vi "MainN.vi"() -> ()   [LabVIEW 2013]
uses:
  ReceiveStrDismantle/MMI_BCM_2A1.ctl
  ReceiveStrDismantle/MMI_AC_2.ctl
  ReceiveStrDismantle/MMI_PEPS_2A7.ctl
  Log.ctl
  SendCmdStr/Input1.ctl
  SendCmdStr/Input2.ctl
  SendCmdStr/HVSM.ctl
  SendCmdStr/TCM.ctl
  SendCmdStr/AC_2F1.ctl
  SendCmdStr/AC_2F2.ctl
  SendCmdStr/BCM_284.ctl
  SendCmdStr/BCM_LDoor_285.ctl
  SendCmdStr/BCM_287.ctl
  SendCmdStr/GW_PEPS_2FC.ctl
  SendCmdStr/TCU_113.ctl
  SendCmdStr/ESC_125.ctl
  SendCmdStr/SAS_0E0.ctl
  SendCmdStr/BCM_Ligh_1F0.ctl
  SendCmdStr/IPK_3F0.ctl
  GlobalVariable.vi
  CAN/ControlCAN.dll
panel:
  in  "刷新":bool
  in  "周期":u32=100
  out "LogEvent":refnum<user-event>
  in  "Input2":T1
  in  "Input1":T2
  in  "Log":T3
  out "消息":string
  in  "接收":bool
  in  "arraylen":u32
  in  "TREvent":T4={"Tx_Or_Rx"=FALSE, "VCI_CAN_OBJ"={"ID"=0, "TimeStamp"=0, "TimeFlag"=0, "SendType"=1, "RemoteFlag"=0, "ExternFlag"=0, "DataLen"=8, 0, 0, 0, 0, 0, 0, 0, 0, 0, 0, 0}, "VCI_CAN_OBJ_N"=[], "Num"=0}
  out "VCI_CAN_STATUS":T5
  in  "界面标识":string="显示界面"
  in  "滤波ID":u32 format="0x%08x"
  in  "滤波":bool
  in  "发送 ID":u32 format="0x%08x"
  in  "一次发送帧数":u32=1
  out "接收缓冲区":u32
  in  "GetStatus":bool
  in  "GetErrorInfo":bool
  in  "Clear Buffer":bool
  in  "Transmit":bool
  in  "数据输入":string
  in  "帧格式":u8(ring) items=["数据帧", "远程帧"]
  in  "帧类型":u8(ring) items=["标准帧", "扩展帧"]
  in  "发送类型":u8(ring) items=["正常发送", "单次发送", "自发自收", "单次自发自收"]
  in  "索引":u32(ring) items=["0", "1", "2", "3", "4", "5", "6", "7", "8"]
  out "CANStartup":bool
  in  "DevOpen":bool
  in  "OpenDevice":bool
  in  "设备类型":u32(ring)=3 items=["PCI5121"=1, "PCI9810"=2, "USBCAN1"=3, "USBCAN2"=4, "PCI9820"=5, "PCI5110"=7, "PC104CAN"=11, "CANETUDP"=12, "PCI9840B"=14, "PC104C2"=15, "PCI9820I"=16, "CANETTCP"=17, "PCIE9221"=24]
  in  "ResetCAN":bool
  in  "StartCAN":bool
  in  "CAN 通道":u32(ring) items=["0", "1"]
  in  "Baud":u32(ring)=11 caption="波特率" items=["5Kbps", "10Kbps", "20Kbps", "40Kbps", "50Kbps", "80Kbps", "100Kbps", "125Kbps", "200Kbps", "250Kbps", "400Kbps", "500Kbps", "666Kbps", "800Kbps", "1000Kbps"]
  in  "模式":u8(ring) items=["正常", "只听"]
  in  "滤波方式":u8(ring)=1 items=["双滤波", "单滤波"]
  in  "BTR1":u8=20 format="0x%02x"
  in  "BTR0":u8 format="0x%02x"
  in  "屏蔽码":u32=4294967295 format="0x%08x"
  in  "验收码":u32 format="0x%08x"
  out "VCI_ERR_INFO":T6 {"ArLost_ErrData" format="%.0x"; "Passive_ErrData2" format="%.0x"; "Passive_ErrData1" format="%.0x"; "Passive_ErrData0" format="%.0x"; "ErrCode" format="%.0x"}
  out "VCI_CAN_OBJ_TN":T7(array[cluster])
  out "VCI_CAN_OBJ_RN":T7(array[cluster])
  out "VCI_INIT_CONFIG":T8={"AccCode"=0, "AccMask"=4294967295, "Reserved"=0, "Filter"=1, "Timing0"=0, "Timing1"=20, "Mode"=0}
  out "VCI_CAN_OBJ_T":T9={"ID"=0, "TimeStamp"=0, "TimeFlag"=0, "SendType"=1, "RemoteFlag"=0, "ExternFlag"=0, "DataLen"=8, 0, 0, 0, 0, 0, 0, 0, 0, 0, 0, 0}
  out "VCI_CAN_OBJ_R":T9={"ID"=0, "TimeStamp"=0, "TimeFlag"=0, "SendType"=1, "RemoteFlag"=0, "ExternFlag"=0, "DataLen"=8, 0, 0, 0, 0, 0, 0, 0, 0, 0, 0, 0}
  in  "多列列表框":i32(listbox)
  in  "退出":bool
  in  "前面板显示":enum32{"接收", "发送", "帮助"}(tab)
  in  "显示信息":T10(tab)
  out "GPS位置信息2":T11
  out "时间显示":string="时间显示"
  out "日":dbl
  out "月":dbl
  out "年":dbl
  out "秒":dbl
  out "分":dbl
  out "时":dbl
  out "GPS位置信息1":T11
  out "BCM":T12 {"语音命令天窗开关" items=["默认", "停止"]; "天窗开度" scale=0.0..100.0; "右后侧车窗开度" scale=0.0..100.0; "左后侧车窗开度" scale=0.0..100.0; "副驾驶侧车窗开度" scale=0.0..100.0; "伴我回家时间" items=["无", "30s", "60s", "90s"]; "门解锁设置应答" items=["无应答", "应答驾驶门解锁", "应答所有门解锁"]; "天窗翘起控制" items=["无", "倾斜翘起", "倾斜关闭"]; "车窗防夹报警" items=["无", "禁止", "启用"]; "日间行车灯" items=["无", "禁止", "启用"]; "智能弯道灯" items=["无", "禁止", "启用"]; "后视镜自动折叠" items=["无", "禁止", "启用"]; "下雨关窗模式" items=["无", "关", "开"]; "设防提示类型" items=["无", "亮灯并鸣笛", "亮灯", "鸣笛"]; "驾驶侧车窗开度" scale=0.0..100.0}
  out "AC空调":T13 {"空气质量弹窗提醒" items=["未按下", "取消提醒"]; "吹风模式请求" items=["Face", "Bilevel", "Foot", "Foot Screen", "Screen", "未设置"]; "鼓风机风速档位" items=["关闭", "风速1", "风速2", "风速3", "风速4", "风速5", "风速6", "风速7", "风速8", "未设置"]; "左侧设定温度显示" scale=17.5..31.5; "驻车空调设置" items=["无", "关闭", "开启"]}
  out "Skin":T14 {"SVA声音报警设置" items=["无请求", "禁止", "启用"]; "IPK-HUD-MMI皮肤联动" items=["联动", "未联动"]; "总里程清零命令" items=["无命令", "清零"]; "指示目的地距离单位" items=["无显示", "Meter", "KiloMeter"]; "MMI激活HUD" items=["无", "未激活", "已激活"]; "皮肤模式" items=["皮肤1", "皮肤2", "皮肤3"]; "方向盘多功能开关模式" items=["MMImode", "IPKmode", "HUDmode"]; "方向盘返回键动作" items=["未按下", "短按", "长按", "长按不松手"]; "方向盘确认键动作" items=["未按下", "短按", "长按", "长按不松手"]; "方向盘下指示键动作" items=["未按下", "短按", "长按", "长按不松手"]; "方向盘上指示键动作" items=["未按下", "短按", "长按", "长按不松手"]; "方向盘左指示键动作" items=["未按下", "短按", "长按", "长按不松手"]; "方向盘右指示键动作" items=["未按下", "短按", "长按", "长按不松手"]}
  out "PEPS":T15 {"任意门开启锁车报警" items=["无请求", "禁止", "启用", "预留"]; "天窗/遮阳帘关闭设置" items=["无请求", "天窗关闭", "遮阳帘关闭", "预留"]; "车窗透气开启设置" items=["无请求", "禁止", "启用", "预留"]; "前雨刮激活后雨刮" items=["无请求", "不激活", "激活", "预留"]; "AVM道路中标定请求" items=["无请求", "开始标定", "预留"]; "自动开关窗设置显示" items=["无请求", "RKE长按控制", "车钥匙控制", "预留"]; "迎宾灯功能开关" items=["无请求", "禁止", "启用", "预留"]; "钥匙忘车内锁车报警" items=["无请求", "禁止", "启用", "预留"]; "AVAS禁用设置" items=["无请求", "禁止", "启用", "预留"]; "电源非OFF锁车报警" items=["无请求", "禁止", "启用", "预留"]; "外后视镜倒车倾斜" items=["无请求", "禁止所有倾斜", "启用驾驶侧", "启用乘客侧", "启用所有侧"]}
  out "智能信号管理":T16 {"下一拥堵路段的长度" scale=0.0..100.0; "距离下一拥堵路段距离" scale=0.0..100.0; "下一路段拥堵等级" items=["正常", "等级1", "等级2", "等级3"]; "当前路段拥堵等级" items=["正常", "等级1", "等级2", "等级3"]; "当前行驶路况" items=["普通路况", "高速路况", "其它"]; "当前拥堵路段剩余长度" scale=0.0..100.0}
  out "PAS_FCS":T17 {"EVA与驾驶模式联动" items=["无联动", "联动", "预留"]; "EVA排气声浪开关" items=["无响应", "开", "关", "预留"]; "iBooster制动模式" items=["NoRequest", "ComfortMode", "SportMode ", "预留"]; "SUM与驾驶模式联动选择" items=["无联动", "联动", "预留"]; "SUM模式选择" items=["No Action", "Confort", "Sport", "预留"]; "泊入功能选择" items=["无按键按下", "水平按下", "垂直按下", "预留"]; "PAS-APA功能确认或关闭" items=["无按键按下", "确认键按下", "终止键按下", "预留"]; "泊入泊出功能选择" items=["未按下", "PSC按下", "POC按下", "预留"]; "环视摄像头功能状态" items=["未激活", "激活", "保持", "失败"]; "导航状态" items=["正常", "失败", "预留"]; "当前所处道路类型" items=["未知", "高速路", "乡道", "国道", "省道", "主干道", "分叉路", "其它"]; "来自地图数据库的限速" scale=0.0..255.0; "前方匝道距离" items=["无匝道", "1000m", "500m", "200m", "预留"]}
  in  "动作输出":T18(tab)
  in  "日":u8
  in  "月":u8
  in  "年":u32
  in  "秒":u8
  in  "分":u8
  in  "时":u8
  in  "时间显示制":u16(ring) items=["24h", "12h"]
  out "时间设置":string="时间设置"
  in  "设置时间":bool
  in  "HVSM远程控制模式与否":bool
  in  "副驾座椅加热状态":u8(ring) items=["关闭", "Level1", "Level2", "Level3", "预留", "错误"]
  in  "司机座椅加热状态":u8(ring) items=["关闭", "Level1", "Level2", "Level3", "预留", "错误"]
  in  "仪表显示档位状态":u16(ring) items=["无显示", "显示P", "显示R", "显示N", "显示D", "显示M1", "显示M2", "显示M3", "显示M4", "显示M5", "显示M6", "显示M7", "显示M1+", "显示M2+", "显示M3+", "显示M4+", "显示M5+", "显示M6+", "显示M2-", "显示M3-", "显示M4-", "显示M5-", "显示M6-", "显示M7-", "无效", "预留"]
  in  "TCU档位模式":u16(ring) items=["未定义", "P", "R", "N", "D", "M", "预留", "无效"]
  in  "方向盘转向标定位":bool
  in  "实际方向盘转向角":dbl(knob)=-780.0 min=-780.0 max=779.9 step=0.1 scale=-780.0..779.9 scale format="%6.1f"
  in  "方向盘转角速度":i32(slide) min=0 max=1016 step=4 scale=0.0..1016.0
  in  "SASFailureStatus":bool
  in  "TCM指示转向灯开关状态":u16(ring) items=["默认", "转左", "转右", "无效"]
  in  "提示HHC功能是否失效":bool
  in  "EPB系统错误指示":bool
  in  "AVH提示状态":u16(ring) items=["关", "介入", "待机", "错误"]
  in  "ESC信号提示ESP失败":bool
  in  "ABS_ESC信号提示车速":dbl(slide) min=0.0 max=491.34 step=0.06 scale=0.0..491.34 scale format="%#_8f"
  in  "ABS_ESC信号提示车速有效性":bool
  in  "空调按键状态":u16(ring) items=["No Press", "Blowup", "BlowDown", "AC Req", "MaxAcReq", "AUTOreq", "DefrostReq", "RearDefReq", "AirDistributionModeReq", "CycleReq", "DualReq", "IONreq", "AqsReq", "LeftTempUp", "LeftTempDown", "RightTempUp", "RightTempDown", "OFF", "KeyBLW"]
  in  "空调按键触摸状态":u16(ring) items=["No Touch", "KeyLeftTemp", "KeyRightTemp", "KeyAUTO", "KeyAC", "KeyBLW+", "KeyBLW-", "KeyMODE", "KeyDEF", "KeyRearDEF", "KeyIntake", "KeyBLW", "Reserved"]
  in  "AC远程控制模式与否":bool
  in  "空调开关按键音":bool
  in  "左侧设定温度":dbl(slide)=17.5 min=17.5 max=31.5 step=0.5 scale=17.5..31.5 scale format="%#_6f"
  in  "空调开启状态":bool
  in  "吹风模式":u16(ring) items=["Face", "Bilevel", "Foot", "FootScreen", "Screen", "预留", "无效"]
  in  "负离子发生器状态":u16(ring) items=["关闭", "开启", "预留", "错误"]
  in  "吹风档位":u16(ring) items=["关闭", "等级1", "等级2", "等级3", "等级4", "等级5", "等级6", "等级7", "等级8", "无效"]
  in  "空气质量传感器请求":bool
  in  "内外循环进气":u16(ring) items=["Fresh", "循环", "保持", "无效"]
  in  "除霜请求状态":bool
  in  "最大制冷请求状态":bool
  in  "空调按键引起弹窗显示":bool
  in  "自动请求状态":bool
  in  "PM2.5是否超标":bool
  in  "AC大气温度传感器合法":bool
  in  "HVAC请求信号开关":bool
  in  "PM2.5传感器工作状态":u16(ring) items=["初始态", "数据收集中", "完成", "关闭"]
  in  "驻车空调状态":u16(ring) items=["关闭", "开启", "预留", "无效"]
  in  "驻车空调失效状态":u16(ring) items=["失效", "未失效", "预留"]
  in  "AC大气温度传感器读数":dbl(slide)=-40.0 min=-40.0 max=60.0 step=0.5 scale=-40.0..60.0 scale format="%#_8f"
  in  "室内空气PM2.5浓度":i32(slide) min=0 max=999 step=1 scale=0.0..999.0
  in  "室外空气PM2.5浓度":i32(slide) min=0 max=999 step=1 scale=0.0..999.0
  in  "室内空气质量等级":u16(ring) items=["Level1", "Level2", "Level3", "Level4", "Level5", "Level6", "预留", "无效"]
  in  "左前门锁状态":u16(ring) items=["未锁", "已锁", "预留", "错误"]
  in  "左后门锁状态":u16(ring) items=["未锁", "已锁", "预留", "错误"]
  in  "车窗防夹报警应答":bool
  in  "后视镜自动折叠应答":bool
  in  "左前门机械钥匙锁止":bool
  in  "BCM提示左后门状态":bool
  in  "BCM提示左前门状态":bool
  in  "左后侧车窗故障状态":bool
  in  "左后侧车窗位置状态":u16(ring) items=["中间位置", "完全打开", "完全关闭", "无效"]
  in  "左后侧车窗运行状态":u16(ring) items=["停止", "手动升窗", "手动降窗", "自动升窗", "自动降窗", "预留"]
  in  "左后侧车窗防夹抑制状态":bool
  in  "左后车窗侧防夹检测":bool
  in  "左后侧车窗开度值":i32(slide) min=0 max=100 step=1 scale=0.0..100.0
  in  "左后侧车窗有效位":bool
  in  "驾驶侧车窗故障状态":bool
  in  "驾驶侧车窗位置状态":u16(ring) items=["中间位置", "完全打开", "完全关闭", "无效"]
  in  "驾驶侧防夹抑制状态":bool
  in  "驾驶侧防夹检测":bool
  in  "驾驶侧车窗有效位":bool
  in  "驾驶侧车窗开度值":i32(slide) min=0 max=100 step=1 scale=0.0..100.0
  in  "驾驶侧车窗运行状态":u16(ring) items=["停止", "手动升窗", "手动降窗", "自动升窗", "自动降窗", "预留"]
  in  "实际天窗位置":u16(ring) items=["位置未知", "完全关闭", "完全打开", "倾斜与张开之间", "完全倾斜", "倾斜与关闭之间", "滑动开启舒适位置", "预留"]
  in  "天窗故障状态":bool
  in  "天窗防夹触发":bool
  in  "天窗有效位":bool
  in  "天窗运行状态":u16(ring) items=["Not Pressed", "Manual slide open", "Manual slide close", "Manual tilt open", "Manual tilt close", "Auto slide open", "Auto slide close", "Auto tilt open", "Auto tilt close", "Moving uninitialized", "Reversing", "Reserved"]
  in  "天窗/遮阳帘关闭反馈":bool
  in  "右前盲区可视按键":bool
  in  "车窗透气反馈":bool
  in  "离合器踏板开关":bool
  in  "BCM电源模式":u16(ring) items=["关闭", "ACC", "开启", "预留", "START"]
  in  "手动车是否挂入倒挡":bool
  in  "前雨刮激活后雨刮":bool
  in  "日间行车灯设置":bool
  in  "设防提示类型设置":u16(ring) items=["无", "亮灯并鸣笛", "亮灯", "鸣笛"]
  in  "智能弯道灯设置":bool
  in  "RLS下雨关窗模式":u16(ring) items=["关", "开", "预留", "错误"]
  in  "雨刮随速功能":bool
  in  "寻车报警类型设置":bool
  in  "防盗报警状态":u16(ring) items=["报警", "预报警", "禁止报警", "提醒", "警报", "部分报警", "未用"]
  in  "自动开关窗设置":u16(ring) items=["禁止", "RKE长按控制", "车钥匙控制", "预留"]
  in  "伴我回家时间选择":u16(ring) items=["无", "30s", "60s", "90s"]
  in  "后除霜开关":bool
  in  "BCM提示引擎盖开关":u16(ring) items=["关闭", "半开", "预留", "无效"]
  in  "后车窗加热器激活":u16(ring) items=["未激活", "激活", "预留", "无效"]
  in  "BCM提示后盖箱开关":bool
  in  "天窗水平开度值":i32(slide) min=0 max=100 step=1 scale=0.0..100.0
  in  "发送机状态信息":u16(ring) items=["Engine Stop", "Cranking", "Stopping", "Running", "Reserved", "Reserved", "Abnormal", "Invalid"]
  in  "BCM提醒用户位置灯状态":bool
  in  "BCM指示转向拔杆状态":u16(ring) items=["Inactive", "Turn left", "Turn right", "Error status"]
  in  "车窗防夹报警设置应答":bool
  in  "任意门开启锁车报警配置":bool
  in  "电源非OFF锁车报警配置":bool
  in  "钥匙忘车内锁车报警配置":bool
  in  "迎宾灯功能开启关闭响应":bool
  in  "GW信号指示PEPS是否超时2":bool
  in  "GW信号指示PEPS是否超时1":bool
  in  "后备箱不带钥匙解锁配置":bool
  in  "PEPS远程在远程模式？":bool
  in  "PEPS电源模式":u16(ring) items=["OFF", "ACC", "ON", "Reserved", "START", "Reserved", "Reserved", "Reserved"]
  in  "PEPS电源模式有效指示":u16(ring) items=["Not available", "Invalid", "Valid", "Reserved"]
  in  "车机设置:1F0":bool
  in  "车机设置:085":bool
  in  "车机设置:2FC":bool
  in  "BCM控制:287":bool
  in  "BCM控制:284":bool
  in  "车身控制车窗:285":bool
  in  "AC控制:2F2":bool
  in  "AC控制:2F1":bool
  in  "ESC控制:125":bool
  in  "TCM开关:281":bool
  in  "SAS转角状态:0E0":bool
  in  "HVSM控制:2C1":bool
  in  "TCU控制:113":bool
  in  "IPK时间:3F0":bool
  in  "ICU":bool
  in  "FCS":bool
  in  "VCU":bool
  in  "OBC":bool
  in  "AVAS":bool
  in  "TBOX":bool
  in  "GW":bool
  in  "PAS":bool
  in  "SAS":bool
  in  "DVR":bool
  in  "BMSH":bool
  # "3E1"
  # "2AF"
  # "3E2"
  # "2A1"
  # "2A5"
  # "2A4"
  # "2A7"
  # "2D0"
  # "2A8"
  # "3F0"
  # "1000ms"
  # "2C1"
  # "100ms"
  # "113"
  # "20ms"
  # "0E0"
  # "10ms"
  # "281"
  # "100ms"
  # "125"
  # "20ms"
  # "2F1"
  # "2F2"
  # "100ms"
  # "100ms"
  # "285"
  # "100ms"
  # "284"
  # "287"
  # "100ms"
  # "100ms"
  # "2FC"
  # "100ms"
  # "1F0"
  # "50ms"
  # "085"
  # "10ms"
  # "ICUMissing：26D"
  # "AVASMissing：2B2"
  # "1000ms"
  # "100ms"
  # "FCSMissing：1B0"
  # "TBOXMissing：292"
  # "100ms"
  # "20ms"
  # "发送控制按钮"
  # "100ms"
  # "100ms"
  # "VCUMissing：162"
  # "GWMissing：2FD"
  # "10ms"
  # "10ms"
  # "OBCMissing：220"
  # "PASMissing：390"
  # "50ms"
  # "100ms"
  # "SASMissing：0E0"
  # "DVRMissing：2B1"
  # "100ms"
  # "20ms"
  # "丢失模拟开关"
  # "100ms"
  # "BMSHMissing：2F4"
  # "100ms"
  # "100ms"
  # "1：启动软件。\n2：选择正确的设备类型（默认为USBCAN1）、波特率（默认值为500K）、\n模式选择正常、索引号通常选0、CAN通道通常选0。周期为帧发送的频次，次数为\n发送帧数据的次数\n3：点击打开设备按钮、其下方绿色显示键点亮，说明打开设备成功，否则弹框\n报错。接下来点击打开CAN按钮，其下方绿色显示键点亮，说明打开CAN通道成功，\n否则弹框报错。\n4：选择相应发送类型（默认为正常发送）、帧类型（默认为标准帧）、帧格式（\n默认为数据帧）。在发送ID中输入数据帧ID（十六进制）、数据输入中输入数据、\n一次发送帧数默认为1、点击发送按键。\n5：菜单栏<界面切换：接收、发送、帮助、关于>\n6：接收是模拟器接收来自车身MMI的数据帧解析显示界面（下部有选项卡）\n7：发送则为模拟器主动向CAN总线中发送CAN数据的界面（下部有选项卡）\n8：关于则为软件一些基本信息\n9：操作发送界面中按键和下拉框前，请确保CAN通道已正常打开！\n10：要周期发送某个ID，先在模拟丢失选项卡处勾选相应ID"
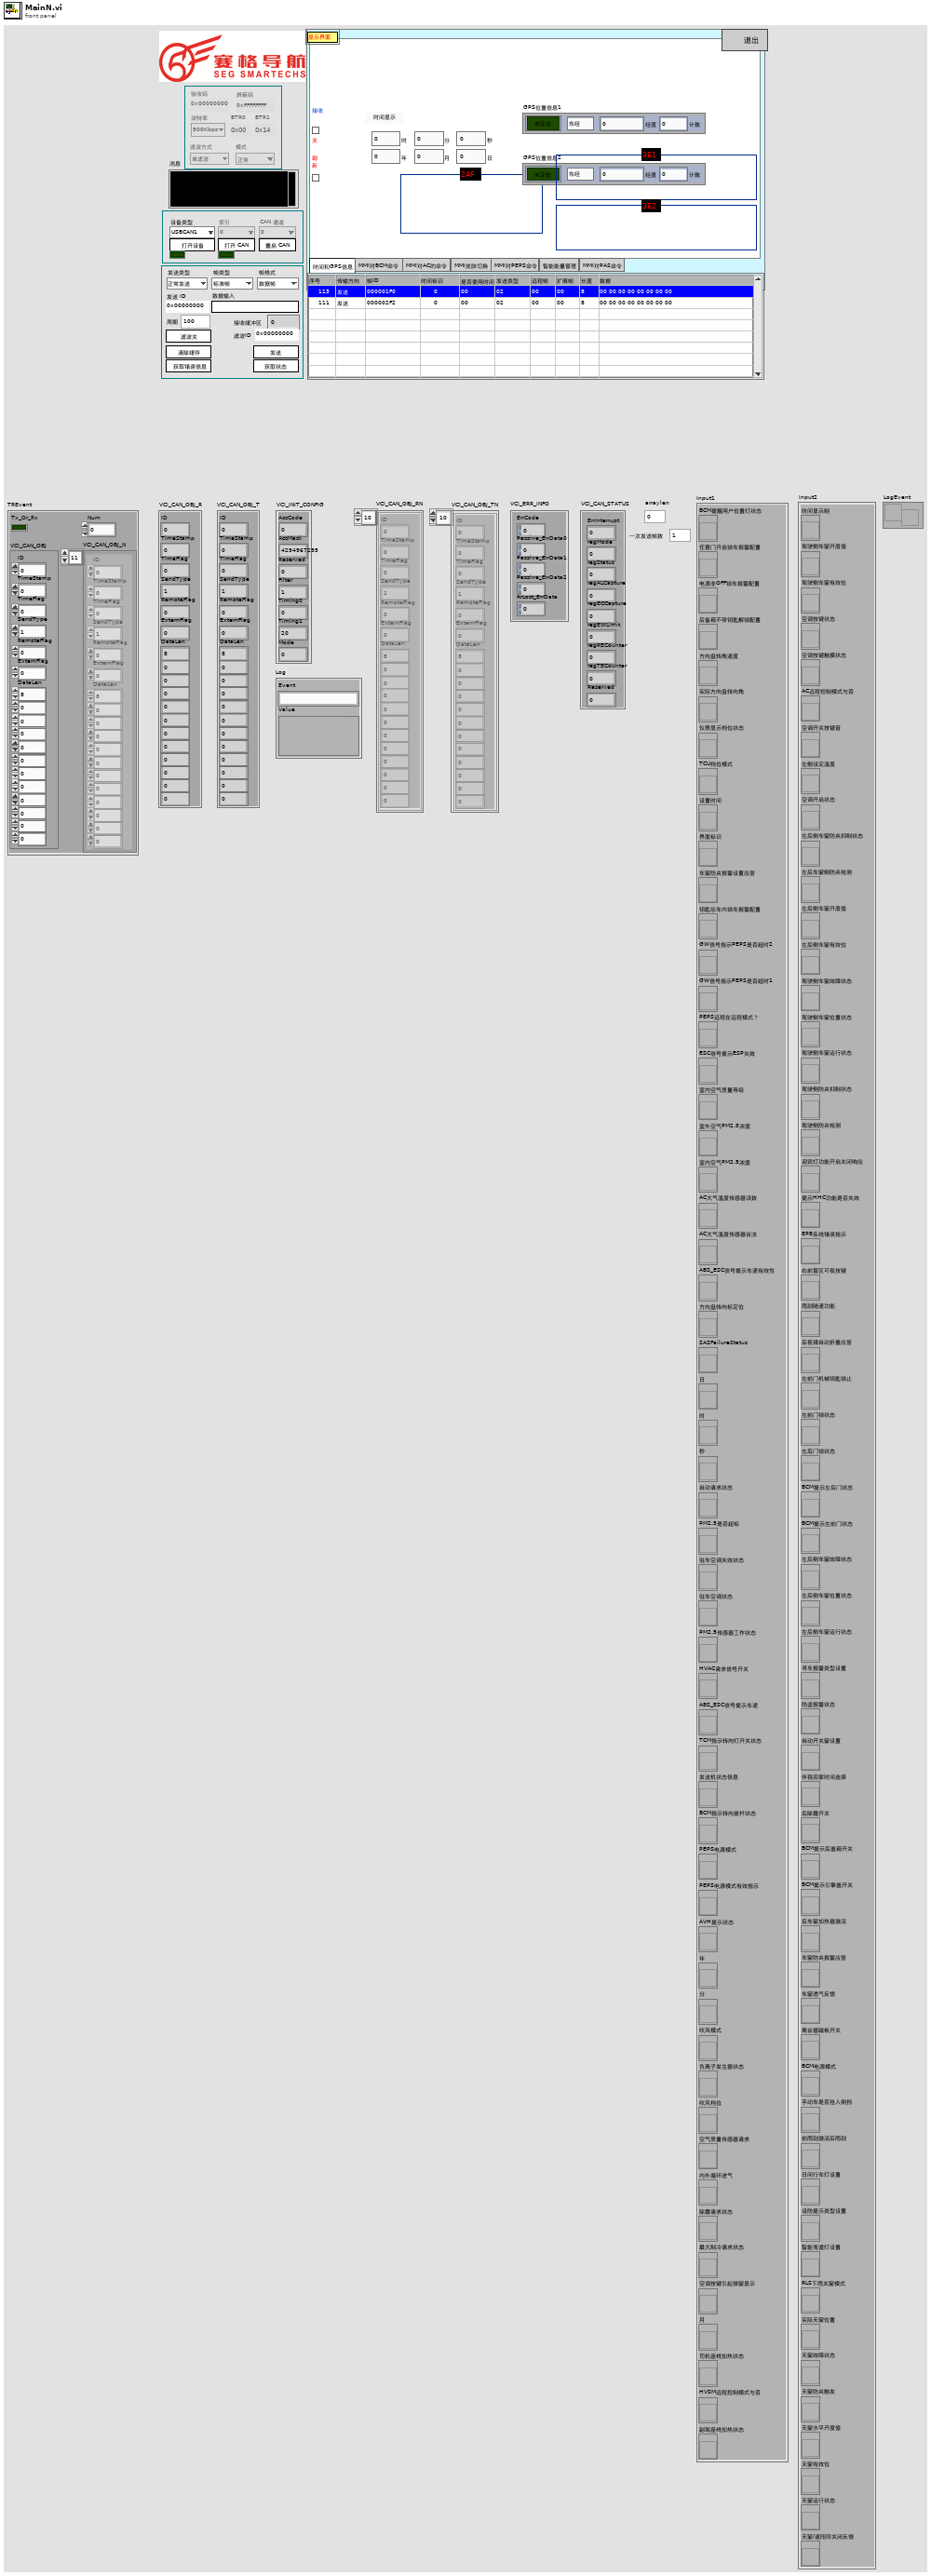
[diagram p1: front panel]
types:
  T1 = typedef "Input2.ctl" = cluster{"时间显示制":refnum<vi>, "驾驶侧车窗开度值":refnum<vi>, "驾驶侧车窗有效位":refnum<vi>, "空调按键状态":refnum<vi>, "空调按键触摸状态":refnum<vi>, "AC远程控制模式与否":refnum<vi>, "空调开关按键音":refnum<vi>, "左侧设定温度":refnum<vi>, "空调开启状态":refnum<vi>, "左后侧车窗防夹抑制状态":refnum<vi>, "左后车窗侧防夹检测":refnum<vi>, "左后侧车窗开度值":refnum<vi>, "左后侧车窗有效位":refnum<vi>, "驾驶侧车窗故障状态":refnum<vi>, "驾驶侧车窗位置状态":refnum<vi>, "驾驶侧车窗运行状态":refnum<vi>, "驾驶侧防夹抑制状态":refnum<vi>, "驾驶侧防夹检测":refnum<vi>, "迎宾灯功能开启关闭响应":refnum<vi>, "提示HHC功能是否失效":refnum<vi>, "EPB系统错误指示":refnum<vi>, "右前盲区可视按键":refnum<vi>, "雨刮随速功能":refnum<vi>, "后视镜自动折叠应答":refnum<vi>, "左前门机械钥匙锁止":refnum<vi>, "左前门锁状态":refnum<vi>, "左后门锁状态":refnum<vi>, "BCM提示左后门状态":refnum<vi>, "BCM提示左前门状态":refnum<vi>, "左后侧车窗故障状态":refnum<vi>, "左后侧车窗位置状态":refnum<vi>, "左后侧车窗运行状态":refnum<vi>, "寻车报警类型设置":refnum<vi>, "防盗报警状态":refnum<vi>, "自动开关窗设置":refnum<vi>, "伴我回家时间选择":refnum<vi>, "后除霜开关":refnum<vi>, "BCM提示后盖箱开关":refnum<vi>, "BCM提示引擎盖开关":refnum<vi>, "后车窗加热器激活":refnum<vi>, "车窗防夹报警应答":refnum<vi>, "车窗透气反馈":refnum<vi>, "离合器踏板开关":refnum<vi>, "BCM电源模式":refnum<vi>, "手动车是否挂入倒挡":refnum<vi>, "前雨刮激活后雨刮":refnum<vi>, "日间行车灯设置":refnum<vi>, "设防提示类型设置":refnum<vi>, "智能弯道灯设置":refnum<vi>, "RLS下雨关窗模式":refnum<vi>, "实际天窗位置":refnum<vi>, "天窗故障状态":refnum<vi>, "天窗防夹触发":refnum<vi>, "天窗水平开度值":refnum<vi>, "天窗有效位":refnum<vi>, "天窗运行状态":refnum<vi>, "天窗/遮阳帘关闭反馈":refnum<vi>}
  T2 = typedef "Input1.ctl" = cluster{"BCM提醒用户位置灯状态":refnum<vi>, "任意门开启锁车报警配置":refnum<vi>, "电源非OFF锁车报警配置":refnum<vi>, "后备箱不带钥匙解锁配置":refnum<vi>, "方向盘转角速度":refnum<vi>, "实际方向盘转向角":refnum<vi>, "仪表显示档位状态":refnum<vi>, "TCU档位模式":refnum<vi>, "设置时间":refnum<vi>, "界面标识":refnum<vi>, "车窗防夹报警设置应答":refnum<vi>, "钥匙忘车内锁车报警配置":refnum<vi>, "GW信号指示PEPS是否超时2":refnum<vi>, "GW信号指示PEPS是否超时1":refnum<vi>, "PEPS远程在远程模式？":refnum<vi>, "ESC信号提示ESP失败":refnum<vi>, "室内空气质量等级":refnum<vi>, "室外空气PM2.5浓度":refnum<vi>, "室内空气PM2.5浓度":refnum<vi>, "AC大气温度传感器读数":refnum<vi>, "AC大气温度传感器合法":refnum<vi>, "ABS_ESC信号提示车速有效性":refnum<vi>, "方向盘转向标定位":refnum<vi>, "SASFailureStatus":refnum<vi>, "日":refnum<vi>, "时":refnum<vi>, "秒":refnum<vi>, "自动请求状态":refnum<vi>, "PM2.5是否超标":refnum<vi>, "驻车空调失效状态":refnum<vi>, "驻车空调状态":refnum<vi>, "PM2.5传感器工作状态":refnum<vi>, "HVAC请求信号开关":refnum<vi>, "ABS_ESC信号提示车速":refnum<vi>, "TCM指示转向灯开关状态":refnum<vi>, "发送机状态信息":refnum<vi>, "BCM指示转向拔杆状态":refnum<vi>, "PEPS电源模式":refnum<vi>, "PEPS电源模式有效指示":refnum<vi>, "AVH提示状态":refnum<vi>, "年":refnum<vi>, "分":refnum<vi>, "吹风模式":refnum<vi>, "负离子发生器状态":refnum<vi>, "吹风档位":refnum<vi>, "空气质量传感器请求":refnum<vi>, "内外循环进气":refnum<vi>, "除霜请求状态":refnum<vi>, "最大制冷请求状态":refnum<vi>, "空调按键引起弹窗显示":refnum<vi>, "月":refnum<vi>, "司机座椅加热状态":refnum<vi>, "HVSM远程控制模式与否":refnum<vi>, "副驾座椅加热状态":refnum<vi>}
  T3 = typedef "Log.ctl" = cluster{"Event":string, "Value":variant}
  T4 = cluster{"Tx_Or_Rx":bool, "VCI_CAN_OBJ":cluster{"ID":u32, "TimeStamp":u32, "TimeFlag":u8, "SendType":u8, "RemoteFlag":u8, "ExternFlag":u8, "DataLen":u8, u8, u8, u8, u8, u8, u8, u8, u8, u8, u8, u8}, "VCI_CAN_OBJ_N":cluster{"ID":u32, "TimeStamp":u32, "TimeFlag":u8, "SendType":u8, "RemoteFlag":u8, "ExternFlag":u8, "DataLen":u8, u8, u8, u8, u8, u8, u8, u8, u8, u8, u8, u8}[], "Num":u32}
  T5 = cluster{"ErrInterrupt":u8, "regMode":u8, "regStatus":u8, "regALCapture":u8, "regECCapture":u8, "regEWLimit":u8, "regRECounter":u8, "regTECounter":u8, "Reserved":u32}
  T6 = cluster{"ErrCode":u32, "Passive_ErrData0":u8, "Passive_ErrData1":u8, "Passive_ErrData2":u8, "ArLost_ErrData":u8}
  T7 = cluster{"ID":u32, "TimeStamp":u32, "TimeFlag":u8, "SendType":u8, "RemoteFlag":u8, "ExternFlag":u8, "DataLen":u8, u8, u8, u8, u8, u8, u8, u8, u8, u8, u8, u8}[]
  T8 = cluster{"AccCode":u32, "AccMask":u32, "Reserved":u32, "Filter":u8, "Timing0":u8, "Timing1":u8, "Mode":u8}
  T9 = cluster{"ID":u32, "TimeStamp":u32, "TimeFlag":u8, "SendType":u8, "RemoteFlag":u8, "ExternFlag":u8, "DataLen":u8, u8, u8, u8, u8, u8, u8, u8, u8, u8, u8, u8}
  T10 = enum32{"时间和GPS信息", "MMI对BCM命令", "MMI对AC的命令", "MMI皮肤切换", "MMI对PEPS命令", "智能能量管理", "MMI对PAS命令"}
  T11 = cluster{"经度":u32, "经度状态":enum16{"东经", "西经"}, "定位状态":bool, "计数":u8}
  T12 = typedef "MMI_BCM_2A1.ctl" = cluster{"设防提示类型":u16, "下雨关窗模式":u16, "后视镜自动折叠":u16, "智能弯道灯":u16, "日间行车灯":u16, "车窗防夹报警":u16, "天窗翘起控制":u16, "门解锁设置应答":u16, "伴我回家时间":u16, "驾驶侧车窗开度":u8, "后除霜按键":bool, "副驾驶侧车窗开度":u8, "左后侧车窗开度":u8, "右后侧车窗开度":u8, "语音命令天窗开关":u16, "天窗开度":u8}
  T13 = typedef "MMI_AC_2.ctl" = cluster{"自动按键":bool, "空调开启按键":bool, "最大制冷按键":bool, "除霜按键":bool, "内外循环按键":bool, "压缩机请求按键":bool, "鼓风机风速档位":u16, "负离子发生器按键":bool, "吹风模式请求":u16, "空调电源按键":bool, "左侧设定温度显示":dbl, "驻车空调设置":u16, "空气质量弹窗提醒":u16}
  T14 = cluster{"方向盘右指示键动作":u16, "方向盘左指示键动作":u16, "方向盘上指示键动作":u16, "方向盘下指示键动作":u16, "方向盘确认键动作":u16, "方向盘返回键动作":u16, "方向盘多功能开关模式":u16, "皮肤模式":u16, "MMI激活HUD":u16, "指示目的地距离单位":u16, "总里程清零命令":u16, "IPK-HUD-MMI皮肤联动":u16, "SVA声音报警设置":u16}
  T15 = typedef "MMI_PEPS_2A7.ctl" = cluster{"外后视镜倒车倾斜":u16, "电源非OFF锁车报警":u16, " 任意门开启锁车报警":u16, "AVAS禁用设置":u16, "钥匙忘车内锁车报警":u16, "迎宾灯功能开关":u16, "自动开关窗设置显示":u16, "AVM道路中标定请求":u16, "前雨刮激活后雨刮":u16, "车窗透气开启设置":u16, "天窗/遮阳帘关闭设置":u16}
  T16 = cluster{"进入智能管理模式":bool, "导航设置成功标识":bool, "当前行驶路况":u16, "当前路段拥堵等级":u16, "当前拥堵路段剩余长度":dbl, "下一路段拥堵等级":u16, "距离下一拥堵路段距离":dbl, "下一拥堵路段的长度":dbl}
  T17 = cluster{"来自地图数据库的限速":i32, " 前方匝道距离":u16, "当前所处道路类型":u16, "导航状态":u16, "指示前方收费站":bool, "环视摄像头功能状态":u16, "泊入泊出功能选择":u16, "PSA-SVA功能输入":bool, "PAS-APA功能确认或关闭":u16, "泊入功能选择":u16, "指示前方隧道":bool, "指示前方目的地":bool, "SUM模式选择":u16, "SUM与驾驶模式联动选择":u16, "EVA排气声浪开关":u16, "EVA与驾驶模式联动":u16, "iBooster制动模式":u16, "消息计数":u8}
  T18 = enum32{"IPK时间", "HVSM控制", "TCU控制", "SAS转角状态", "TCM开关", "ESC控制", "AC控制", "车身控制车窗", "BCM控制", "车机设置", "模拟丢失"}
  T19 = typedef "IPK_3F0.ctl" = cluster{"秒":u8, "分":u8, "时":u8, "时间显示制":u16, "日":u8, "月":u8, "年":u8}
  T20 = typedef "BCM_Ligh_1F0.ctl" = cluster{"车窗防夹报警设置应答":bool, "BCM指示转向拔杆状态":u16, "BCM提醒用户位置灯状态":bool}
  T21 = typedef "SAS_0E0.ctl" = cluster{"实际方向盘转向角":dbl, "方向盘转角速度":i32, "方向盘转向标定位":bool, "SASFailureStatus":bool, "计数":u8}
  T22 = typedef "ESC_125.ctl" = cluster{"ESC信号提示ESP失败":bool, "ABS_ESC信号提示车速有效性":bool, "ABS_ESC信号提示车速":dbl, "AVH提示状态":u16, "EPB系统错误指示":bool, "提示HHC功能是否失效":bool}
  T23 = typedef "TCU_113.ctl" = cluster{"TCU档位模式":u8, "仪表显示档位状态":u8}
  T24 = typedef "GW_PEPS_2FC.ctl" = cluster{"PEPS电源模式有效指示":u16, "PEPS电源模式":u16, "PEPS远程在远程模式？":bool, "后备箱不带钥匙解锁配置":bool, "GW信号指示PEPS是否超时1":bool, "GW信号指示PEPS是否超时2":bool, "迎宾灯功能开启关闭响应":bool, "钥匙忘车内锁车报警配置":bool, "电源非OFF锁车报警配置":bool, "任意门开启锁车报警配置":bool}
  T25 = typedef "BCM_287.ctl" = cluster{"天窗运行状态":u16, "天窗有效位":bool, "天窗水平开度值":i32, "天窗防夹触发":bool, "天窗故障状态":bool, "实际天窗位置":u16}
  T26 = typedef "BCM_LDoor_285.ctl" = cluster{"驾驶侧车窗有效位":bool, "驾驶侧车窗开度值":i32, "驾驶侧防夹检测":bool, "驾驶侧防夹抑制状态":bool, "驾驶侧车窗运行状态":u16, "驾驶侧车窗位置状态":u16, "驾驶侧车窗故障状态":bool, "左后侧车窗有效位":bool, "左后侧车窗开度值":i32, "左后车窗侧防夹检测":bool, "左后侧车窗防夹抑制状态":bool, "左后侧车窗运行状态":u16, "左后侧车窗位置状态":u16, "左后侧车窗故障状态":bool, "BCM提示左前门状态":bool, "BCM提示左后面状态":bool, "左后门锁状态":u16, "左前门锁状态":u16, "左前门机械钥匙锁止":bool, "后视镜自动折叠应答":bool, "车窗防夹报警应答":bool}
  T27 = typedef "BCM_284.ctl" = cluster{"后车窗加热器激活":u16, "BCM提示引擎盖开关":u16, "BCM提示后盖箱开关":bool, "后除霜开关":bool, "伴我回家时间选择":u16, "自动开关窗设置":u16, "防盗报警状态":u16, "寻车报警类型设置":bool, "雨刮随速功能":bool, "RLS下雨关窗模式":u16, "智能弯道灯设置":bool, "设防提示类型设置":u16, "日间行车灯设置":bool, "前雨刮激活后雨刮":bool, "手动车是否挂入倒挡":bool, "BCM电源模式":u16, "离合器踏板开关":bool, "车窗透气反馈":bool, "右前盲区可视按键":bool, "天窗/遮阳帘关闭反馈":bool}
  T28 = typedef "AC_2F2.ctl" = cluster{"自动请求状态":bool, "空调按键引起弹窗显示":bool, "最大制冷请求状态":bool, "除霜请求状态":bool, "内外循环进气":u16, "空气质量传感器请求":bool, "吹风档位":u16, "负离子发生器状态":u16, "吹风模式":u16, "空调开启状态":bool, "左侧设定温度":dbl, "空调开关按键音":bool, "AC远程控制模式与否":bool, "空调按键触摸状态":u16, "空调按键状态":u16}
  T29 = typedef "AC_2F1.ctl" = cluster{"HVAC请求信号开关":bool, "AC大气温度传感器合法":bool, "AC大气温度传感器读数":dbl, "室内空气PM2.5浓度":i32, "室外空气PM2.5浓度":i32, "室内空气质量等级":u16, "PM2.5传感器工作状态":u16, "驻车空调状态":u16, "驻车空调失效状态":u16, "PM2.5是否超标":bool}
  T30 = typedef "TCM.ctl" = cluster{"TCM指示转向灯开关状态":u16, "计数":u8}
  T31 = typedef "HVSM.ctl" = cluster{"司机座椅加热状态":u8, "副驾座椅加热状态":u8, "HVSM远程控制模式":bool}
  T32 = cluster{"事件注册引用句柄":refnum<event-registration>, "事件注册引用句柄":refnum<event-registration>}
  T33 = cluster{bool, "VCI_CAN_OBJ_T":cluster{"ID":u32, "TimeStamp":u32, "TimeFlag":u8, "SendType":u8, "RemoteFlag":u8, "ExternFlag":u8, "DataLen":u8, u8, u8, u8, u8, u8, u8, u8, u8, u8, u8, u8}, "VCI_CAN_OBJ_RN":cluster{"ID":u32, "TimeStamp":u32, "TimeFlag":u8, "SendType":u8, "RemoteFlag":u8, "ExternFlag":u8, "DataLen":u8, u8, u8, u8, u8, u8, u8, u8, u8, u8, u8, u8}[], "return type":u32}
  T34 = cluster{"秒":i32, "分":i32, "时":i32, "日":i32, "月":i32, "年":i32}
  T35 = cluster{"设防提示类型":u16, "下雨关窗模式":u16, "后视镜自动折叠":u16, "智能弯道灯":u16, "日间行车灯":u16, "车窗防夹报警":u16, "天窗翘起控制":u16, "门解锁设置应答":u16, "伴我回家时间":u16, "驾驶侧车窗开度":u8, "后除霜按键":bool, "副驾驶侧车窗开度":u8, "左后侧车窗开度":u8, "右后侧车窗开度":u8, "语音命令天窗开关":u16, "天窗开度":u8}
  T36 = cluster{"自动按键":bool, "空调开启按键":bool, "最大制冷按键":bool, "除霜按键":bool, "内外循环按键":bool, "压缩机请求按键":bool, "鼓风机风速档位":u16, "负离子发生器按键":bool, "吹风模式请求":u16, "空调电源按键":bool, "左侧设定温度":dbl, "驻车空调设置":u16, "空气质量弹窗提醒":u16}
  T37 = cluster{"外后视镜倒车倾斜":u16, "电源非OFF锁车报警":u16, " 任意门开启锁车报警":u16, "AVAS禁用设置":u16, "钥匙忘车内锁车报警":u16, "迎宾灯功能开关":u16, "自动开关窗设置":u16, "AVM道路中标定请求":u16, "前雨刮激活后雨刮":u16, "车窗透气开启设置":u16, "天窗/遮阳帘关闭设置":u16}
  T38 = cluster{"进入智能管理模式":bool, "导航设置成功标识":bool, "当前行驶路况":u16, "当前路段拥堵等级":u16, "当前拥堵路段剩余长度":i32, "下一路段拥堵等级":u16, "距离下一拥堵路段距离":dbl, "下一拥堵路段的长度":dbl}
  T39 = enum8{"Enabled", "Disabled", "Disabled and Grayed Out"}
  T40 = cluster{"验收码":u32, "屏蔽码":u32, i32, "滤波方式":u8, "BTR0":u8, "BTR1":u8, "模式":u8}
  T41 = cluster{"[0]":u32, "[1]":u32, "[2]":u32, "[3]":u32, "[4]":u32, "[5]":u32, "[6]":u32, "[7]":u32, "[8]":u32}
  T42 = cluster{"发送 ID":u32, u32, u8, "发送类型":u8, "帧格式":u8, "帧类型":u8, i32, "[0]":u32, "[1]":u32, "[2]":u32, "[3]":u32, "[4]":u32, "[5]":u32, "[6]":u32, "[7]":u32, u32, u32, u32}
  T43 = cluster{bool, "VCI_CAN_OBJ_R":cluster{"ID":u32, "TimeStamp":u32, "TimeFlag":u8, "SendType":u8, "RemoteFlag":u8, "ExternFlag":u8, "DataLen":u8, u8, u8, u8, u8, u8, u8, u8, u8, u8, u8, u8}, "pReceive":cluster{"ID":u32, "TimeStamp":u32, "TimeFlag":u8, "SendType":u8, "RemoteFlag":u8, "ExternFlag":u8, "DataLen":u8, u8, u8, u8, u8, u8, u8, u8, u8, u8, u8, u8}[], "return type":u32}
  T44 = enum32{"invalid app kind", "Development System", "Run Time System", "Student Edition", "Embedded LabVIEW", "Evaluation", "Custom"}
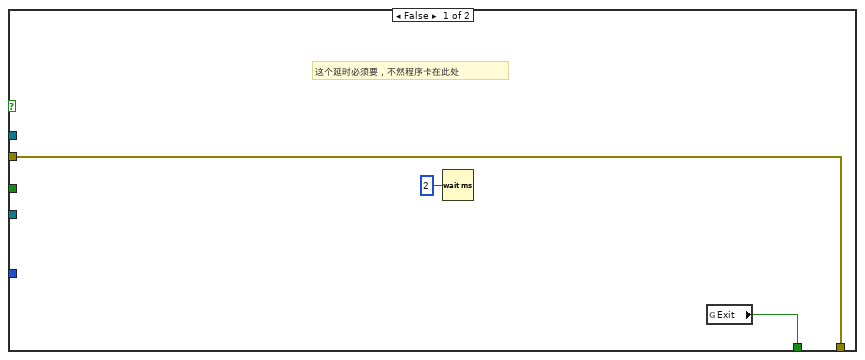
[diagram p2: hidden frame]
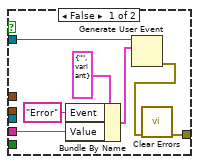
[diagram p5: hidden frame]
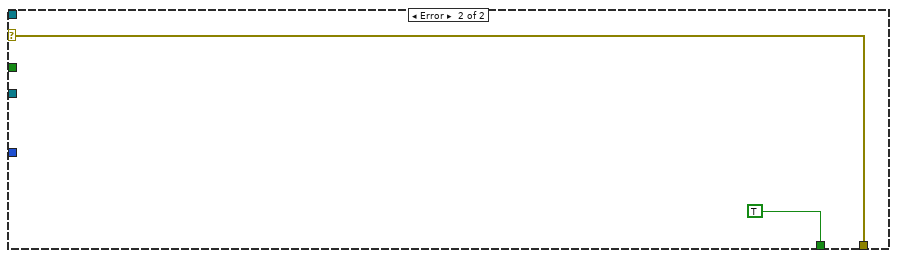
[diagram p6: hidden frame]
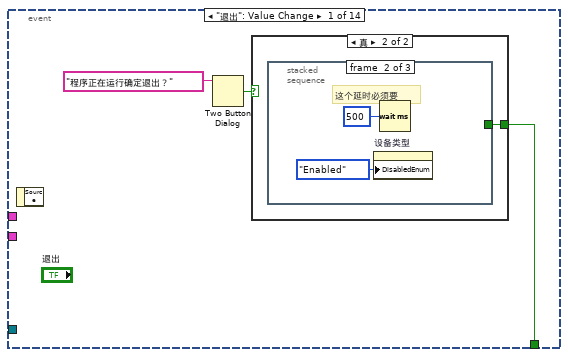
[diagram p7: hidden frame]
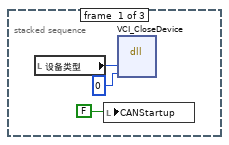
[diagram p9: hidden frame]
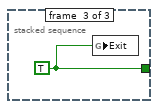
[diagram p10: hidden frame]
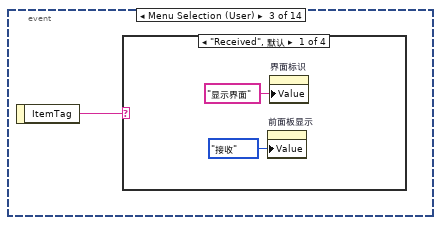
[diagram p12: hidden frame]
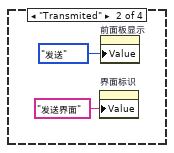
[diagram p13: hidden frame]
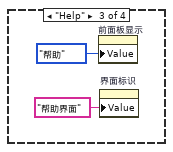
[diagram p14: hidden frame]
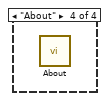
[diagram p15: hidden frame]
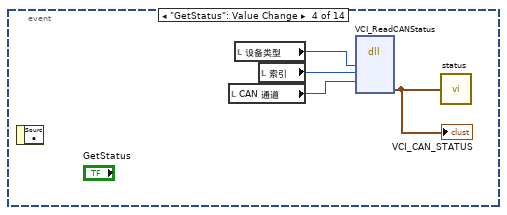
[diagram p16: hidden frame]
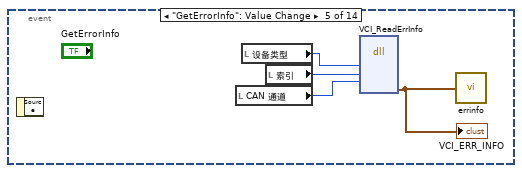
[diagram p17: hidden frame]
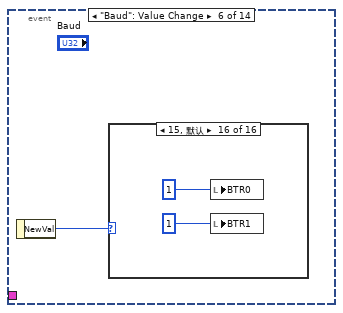
[diagram p18: hidden frame]
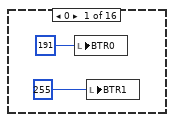
[diagram p19: hidden frame]
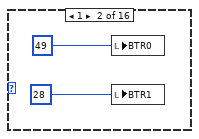
[diagram p20: hidden frame]
diagram:
  n1 = stacked-sequence {
    tunnel: [_ _ _ w172] -> w34
    tunnel: [_ _ _ w190] -> w6
    tunnel: [_ _ _ w168] -> w7
    tunnel: [_ _ _ w171] -> w5
    tunnel: [_ _ w98 _] -> w3
    tunnel: [_ w35 _ _] -> w8
    tunnel: [_ _ _ w165] -> w10
    tunnel: [_ _ _ w160] -> w9
    frame #0 {
    }
    frame #1 {
      n2 = flat-sequence {
        tunnel: [w93] -> w36
        frame #0 {
          # "这个一定要慎重使用，一定放在最前"
          n3 = invoke class="VI" method="Default Vals.Reinit All"() -> (error out=w95:errorcluster)  [unwired: 3 in, 2 out]
          n4 = property on="多列列表框" class="MCListbox (严格)"(error in=w95, "ColHdrString"=string[] ["序号", "传输方向", "帧ID", "时间标识", "是否使用时间标识", "发送类型", "远程帧", "扩展帧", "长度", "数据"] ("列首字符串[]")) -> (error out=w93:errorcluster)  [unwired: 1 in, 1 out]
        }
      }
      n5 = flat-sequence {
        tunnel: w36 -> [_]
        tunnel: [w41] -> w35
        frame #0 {
          n6 = control-ref of="BCM提醒用户位置灯状态"() -> (w92:refnum<vi>)
          n7 = control-ref of="任意门开启锁车报警配置"() -> (w91:refnum<vi>)
          n8 = control-ref of="电源非OFF锁车报警配置"() -> (w90:refnum<vi>)
          n9 = control-ref of="后备箱不带钥匙解锁配置"() -> (w89:refnum<vi>)
          n10 = control-ref of="方向盘转角速度"() -> (w88:refnum<vi>)
          n11 = control-ref of="实际方向盘转向角"() -> (w87:refnum<vi>)
          n12 = control-ref of="仪表显示档位状态"() -> (w86:refnum<vi>)
          n13 = control-ref of="TCU档位模式"() -> (w85:refnum<vi>)
          n14 = control-ref of="设置时间"() -> (w84:refnum<vi>)
          n15 = control-ref of="界面标识"() -> (w83:refnum<vi>)
          n16 = control-ref of="车窗防夹报警设置应答"() -> (w82:refnum<vi>)
          n17 = control-ref of="钥匙忘车内锁车报警配置"() -> (w81:refnum<vi>)
          n18 = control-ref of="GW信号指示PEPS是否超时2"() -> (w80:refnum<vi>)
          n19 = control-ref of="GW信号指示PEPS是否超时1"() -> (w79:refnum<vi>)
          n20 = control-ref of="PEPS远程在远程模式？"() -> (w78:refnum<vi>)
          n21 = control-ref of="ESC信号提示ESP失败"() -> (w77:refnum<vi>)
          n22 = control-ref of="室内空气质量等级"() -> (w76:refnum<vi>)
          n23 = control-ref of="室外空气PM2.5浓度"() -> (w75:refnum<vi>)
          n24 = control-ref of="室内空气PM2.5浓度"() -> (w74:refnum<vi>)
          n25 = control-ref of="AC大气温度传感器读数"() -> (w73:refnum<vi>)
          n26 = control-ref of="AC大气温度传感器合法"() -> (w72:refnum<vi>)
          n27 = control-ref of="ABS_ESC信号提示车速有效性"() -> (w71:refnum<vi>)
          n28 = control-ref of="方向盘转向标定位"() -> (w70:refnum<vi>)
          n29 = control-ref of="SASFailureStatus"() -> (w69:refnum<vi>)
          n30 = control-ref of="日"() -> (w68:refnum<vi>)
          n31 = control-ref of="时"() -> (w67:refnum<vi>)
          n32 = control-ref of="秒"() -> (w66:refnum<vi>)
          n33 = control-ref of="自动请求状态"() -> (w65:refnum<vi>)
          n34 = control-ref of="PM2.5是否超标"() -> (w64:refnum<vi>)
          n35 = control-ref of="驻车空调失效状态"() -> (w63:refnum<vi>)
          n36 = control-ref of="驻车空调状态"() -> (w62:refnum<vi>)
          n37 = control-ref of="PM2.5传感器工作状态"() -> (w61:refnum<vi>)
          n38 = control-ref of="HVAC请求信号开关"() -> (w60:refnum<vi>)
          n39 = control-ref of="ABS_ESC信号提示车速"() -> (w59:refnum<vi>)
          n40 = control-ref of="TCM指示转向灯开关状态"() -> (w58:refnum<vi>)
          n41 = control-ref of="发送机状态信息"() -> (w57:refnum<vi>)
          n42 = control-ref of="BCM指示转向拔杆状态"() -> (w56:refnum<vi>)
          n43 = control-ref of="PEPS电源模式"() -> (w55:refnum<vi>)
          n44 = control-ref of="PEPS电源模式有效指示"() -> (w54:refnum<vi>)
          n45 = control-ref of="AVH提示状态"() -> (w53:refnum<vi>)
          n46 = control-ref of="年"() -> (w52:refnum<vi>)
          n47 = control-ref of="分"() -> (w51:refnum<vi>)
          n48 = control-ref of="吹风模式"() -> (w50:refnum<vi>)
          n49 = control-ref of="负离子发生器状态"() -> (w49:refnum<vi>)
          n50 = control-ref of="吹风档位"() -> (w48:refnum<vi>)
          n51 = control-ref of="空气质量传感器请求"() -> (w47:refnum<vi>)
          n52 = control-ref of="内外循环进气"() -> (w46:refnum<vi>)
          n53 = control-ref of="除霜请求状态"() -> (w45:refnum<vi>)
          n54 = control-ref of="最大制冷请求状态"() -> (w44:refnum<vi>)
          n55 = control-ref of="空调按键引起弹窗显示"() -> (w43:refnum<vi>)
          n56 = control-ref of="月"() -> (w42:refnum<vi>)
          n57 = control-ref of="司机座椅加热状态"() -> (w40:refnum<vi>)
          n58 = control-ref of="HVSM远程控制模式与否"() -> (w39:refnum<vi>)
          n59 = control-ref of="副驾座椅加热状态"() -> (w38:refnum<vi>)
          n60 = Bundle By Name(cluster="Input1", "BCM提醒用户位置灯状态"=w92, "任意门开启锁车报警配置"=w91, "电源非OFF锁车报警配置"=w90, "后备箱不带钥匙解锁配置"=w89, "方向盘转角速度"=w88, "实际方向盘转向角"=w87, "仪表显示档位状态"=w86, "TCU档位模式"=w85, "设置时间"=w84, "界面标识"=w83, "车窗防夹报警设置应答"=w82, "钥匙忘车内锁车报警配置"=w81, "GW信号指示PEPS是否超时2"=w80, "GW信号指示PEPS是否超时1"=w79, "PEPS远程在远程模式？"=w78, "ESC信号提示ESP失败"=w77, "室内空气质量等级"=w76, "室外空气PM2.5浓度"=w75, "室内空气PM2.5浓度"=w74, "AC大气温度传感器读数"=w73, "AC大气温度传感器合法"=w72, "ABS_ESC信号提示车速有效性"=w71, "方向盘转向标定位"=w70, "SASFailureStatus"=w69, "日"=w68, "时"=w67, "秒"=w66, "自动请求状态"=w65, "PM2.5是否超标"=w64, "驻车空调失效状态"=w63, "驻车空调状态"=w62, "PM2.5传感器工作状态"=w61, "HVAC请求信号开关"=w60, "ABS_ESC信号提示车速"=w59, "TCM指示转向灯开关状态"=w58, "发送机状态信息"=w57, "BCM指示转向拔杆状态"=w56, "PEPS电源模式"=w55, "PEPS电源模式有效指示"=w54, "AVH提示状态"=w53, "年"=w52, "分"=w51, "吹风模式"=w50, "负离子发生器状态"=w49, "吹风档位"=w48, "空气质量传感器请求"=w47, "内外循环进气"=w46, "除霜请求状态"=w45, "最大制冷请求状态"=w44, "空调按键引起弹窗显示"=w43, "月"=w42, "司机座椅加热状态"=w40, "HVSM远程控制模式与否"=w39, "副驾座椅加热状态"=w38) -> (w41:T2)
        }
      }
    }
    frame #2 {
      w96 = 0
      w97 = 0
      n61 = control-ref of="时间显示制"() -> (w155:refnum<vi>)
      n62 = control-ref of="驾驶侧车窗开度值"() -> (w154:refnum<vi>)
      n63 = control-ref of="驾驶侧车窗有效位"() -> (w153:refnum<vi>)
      n64 = control-ref of="空调按键状态"() -> (w152:refnum<vi>)
      n65 = control-ref of="空调按键触摸状态"() -> (w151:refnum<vi>)
      n66 = control-ref of="AC远程控制模式与否"() -> (w150:refnum<vi>)
      n67 = control-ref of="空调开关按键音"() -> (w149:refnum<vi>)
      n68 = control-ref of="左侧设定温度"() -> (w148:refnum<vi>)
      n69 = control-ref of="空调开启状态"() -> (w147:refnum<vi>)
      n70 = control-ref of="左后侧车窗防夹抑制状态"() -> (w146:refnum<vi>)
      n71 = control-ref of="左后车窗侧防夹检测"() -> (w145:refnum<vi>)
      n72 = control-ref of="左后侧车窗开度值"() -> (w144:refnum<vi>)
      n73 = control-ref of="左后侧车窗有效位"() -> (w143:refnum<vi>)
      n74 = control-ref of="驾驶侧车窗故障状态"() -> (w142:refnum<vi>)
      n75 = control-ref of="驾驶侧车窗位置状态"() -> (w141:refnum<vi>)
      n76 = control-ref of="驾驶侧车窗运行状态"() -> (w140:refnum<vi>)
      n77 = control-ref of="驾驶侧防夹抑制状态"() -> (w139:refnum<vi>)
      n78 = control-ref of="驾驶侧防夹检测"() -> (w138:refnum<vi>)
      n79 = control-ref of="迎宾灯功能开启关闭响应"() -> (w137:refnum<vi>)
      n80 = control-ref of="提示HHC功能是否失效"() -> (w136:refnum<vi>)
      n81 = control-ref of="EPB系统错误指示"() -> (w135:refnum<vi>)
      n82 = control-ref of="右前盲区可视按键"() -> (w134:refnum<vi>)
      n83 = control-ref of="雨刮随速功能"() -> (w133:refnum<vi>)
      n84 = control-ref of="后视镜自动折叠应答"() -> (w132:refnum<vi>)
      n85 = control-ref of="左前门机械钥匙锁止"() -> (w131:refnum<vi>)
      n86 = control-ref of="左前门锁状态"() -> (w130:refnum<vi>)
      n87 = control-ref of="左后门锁状态"() -> (w129:refnum<vi>)
      n88 = control-ref of="BCM提示左后门状态"() -> (w128:refnum<vi>)
      n89 = control-ref of="BCM提示左前门状态"() -> (w127:refnum<vi>)
      n90 = control-ref of="左后侧车窗故障状态"() -> (w126:refnum<vi>)
      n91 = control-ref of="左后侧车窗位置状态"() -> (w125:refnum<vi>)
      n92 = control-ref of="左后侧车窗运行状态"() -> (w124:refnum<vi>)
      n93 = control-ref of="寻车报警类型设置"() -> (w123:refnum<vi>)
      n94 = control-ref of="防盗报警状态"() -> (w122:refnum<vi>)
      n95 = control-ref of="自动开关窗设置"() -> (w121:refnum<vi>)
      n96 = control-ref of="伴我回家时间选择"() -> (w120:refnum<vi>)
      n97 = control-ref of="后除霜开关"() -> (w119:refnum<vi>)
      n98 = control-ref of="BCM提示后盖箱开关"() -> (w118:refnum<vi>)
      n99 = control-ref of="BCM提示引擎盖开关"() -> (w117:refnum<vi>)
      n100 = control-ref of="后车窗加热器激活"() -> (w116:refnum<vi>)
      n101 = control-ref of="车窗防夹报警应答"() -> (w115:refnum<vi>)
      n102 = control-ref of="车窗透气反馈"() -> (w114:refnum<vi>)
      n103 = control-ref of="离合器踏板开关"() -> (w113:refnum<vi>)
      n104 = control-ref of="BCM电源模式"() -> (w112:refnum<vi>)
      n105 = control-ref of="手动车是否挂入倒挡"() -> (w111:refnum<vi>)
      n106 = control-ref of="前雨刮激活后雨刮"() -> (w110:refnum<vi>)
      n107 = control-ref of="日间行车灯设置"() -> (w109:refnum<vi>)
      n108 = control-ref of="设防提示类型设置"() -> (w108:refnum<vi>)
      n109 = control-ref of="智能弯道灯设置"() -> (w107:refnum<vi>)
      n110 = control-ref of="RLS下雨关窗模式"() -> (w106:refnum<vi>)
      n111 = control-ref of="实际天窗位置"() -> (w105:refnum<vi>)
      n112 = control-ref of="天窗故障状态"() -> (w104:refnum<vi>)
      n113 = control-ref of="天窗防夹触发"() -> (w103:refnum<vi>)
      n114 = control-ref of="天窗水平开度值"() -> (w102:refnum<vi>)
      n115 = control-ref of="天窗有效位"() -> (w101:refnum<vi>)
      n116 = control-ref of="天窗运行状态"() -> (w100:refnum<vi>)
      n117 = control-ref of="天窗/遮阳帘关闭反馈"() -> (w99:refnum<vi>)
      n118 = Bundle By Name(cluster="Input2", "时间显示制"=w155, "驾驶侧车窗开度值"=w154, "驾驶侧车窗有效位"=w153, "空调按键状态"=w152, "空调按键触摸状态"=w151, "AC远程控制模式与否"=w150, "空调开关按键音"=w149, "左侧设定温度"=w148, "空调开启状态"=w147, "左后侧车窗防夹抑制状态"=w146, "左后车窗侧防夹检测"=w145, "左后侧车窗开度值"=w144, "左后侧车窗有效位"=w143, "驾驶侧车窗故障状态"=w142, "驾驶侧车窗位置状态"=w141, "驾驶侧车窗运行状态"=w140, "驾驶侧防夹抑制状态"=w139, "驾驶侧防夹检测"=w138, "迎宾灯功能开启关闭响应"=w137, "提示HHC功能是否失效"=w136, "EPB系统错误指示"=w135, "右前盲区可视按键"=w134, "雨刮随速功能"=w133, "后视镜自动折叠应答"=w132, "左前门机械钥匙锁止"=w131, "左前门锁状态"=w130, "左后门锁状态"=w129, "BCM提示左后门状态"=w128, "BCM提示左前门状态"=w127, "左后侧车窗故障状态"=w126, "左后侧车窗位置状态"=w125, "左后侧车窗运行状态"=w124, "寻车报警类型设置"=w123, "防盗报警状态"=w122, "自动开关窗设置"=w121, "伴我回家时间选择"=w120, "后除霜开关"=w119, "BCM提示后盖箱开关"=w118, "BCM提示引擎盖开关"=w117, "后车窗加热器激活"=w116, "车窗防夹报警应答"=w115, "车窗透气反馈"=w114, "离合器踏板开关"=w113, "BCM电源模式"=w112, "手动车是否挂入倒挡"=w111, "前雨刮激活后雨刮"=w110, "日间行车灯设置"=w109, "设防提示类型设置"=w108, "智能弯道灯设置"=w107, "RLS下雨关窗模式"=w106, "实际天窗位置"=w105, "天窗故障状态"=w104, "天窗防夹触发"=w103, "天窗水平开度值"=w102, "天窗有效位"=w101, "天窗运行状态"=w100, "天窗/遮阳帘关闭反馈"=w99) -> (w98:T1)
      n119 = property on="设备类型" class="Ring (严格)"("DisabledEnum"=w97) -> ()  [unwired: 2 in, 2 out]
      n120 = property on="验收码" class="DigNum (严格)"("DisabledEnum"=w97) -> ()  [unwired: 2 in, 2 out]
      n121 = property on="屏蔽码" class="DigNum (严格)"("DisabledEnum"=w97) -> ()  [unwired: 2 in, 2 out]
      n122 = property on="滤波方式" class="Ring (严格)"("DisabledEnum"=w97) -> ()  [unwired: 2 in, 2 out]
      n123 = property on="索引" class="Ring (严格)"("DisabledEnum"=w97) -> ()  [unwired: 2 in, 2 out]
      n124 = property on="消息" class="Str"("Text.TextColor"=u32 16711680) -> ()  [unwired: 2 in, 2 out]
      n125 = property on="Baud" class="Ring (严格)"("DisabledEnum"=w96) -> ()  [unwired: 2 in, 2 out]
      n126 = property on="BTR0" class="DigNum (严格)"("DisabledEnum"=w96) -> ()  [unwired: 2 in, 2 out]
      n127 = property on="BTR1" class="DigNum (严格)"("DisabledEnum"=w96) -> ()  [unwired: 2 in, 2 out]
      n128 = property on="模式" class="Ring (严格)"("DisabledEnum"=w96) -> ()  [unwired: 2 in, 2 out]
      n129 = property on="CAN 通道" class="Ring (严格)"("DisabledEnum"=w96) -> ()  [unwired: 2 in, 2 out]
    }
    frame #3 {
      w167 = 0
      w185 = u32 10
      w164 = FALSE
      w193 = 2
      n130 = local read "VCI_CAN_OBJ_R"() -> (w189:T9)
      n131 = local read "VCI_CAN_OBJ_T"() -> (w186:T9)
      n132 = property on="OpenDevice" class="Bool (严格)"("DisabledEnum"=w167) -> ()  [unwired: 2 in, 2 out]
      n133 = property on="StartCAN" class="Bool (严格)"("DisabledEnum"=w167) -> ()  [unwired: 2 in, 2 out]
      n134 = property on="ResetCAN" class="Bool (严格)"("DisabledEnum"=w167) -> ()  [unwired: 2 in, 2 out]
      n135 = property on="滤波ID" class="DigNum (严格)"("DisabledEnum"=w167) -> ()  [unwired: 2 in, 2 out]
      n136 = Initialize Array(w189, w185) -> (w188:T7)
      n137 = Initialize Array(w186, w185) -> (w187:T7)
      n138 = property on="前面板显示" class="TabCtl (严格)"("Value"=enum32{"接收", "发送", "帮助"}."发送" ("前面板显示")) -> (error out=w163:errorcluster)  [unwired: 2 in, 1 out]
      n139 = local write "数据输入"("11 22 33 44 55 66 77 88") -> ()
      n140 = local write "arraylen"(w185) -> ()
      n141 = local write "VCI_CAN_OBJ_RN"(w188) -> ()
      n142 = local write "VCI_CAN_OBJ_TN"(w187) -> ()
      n143 = property on="动作输出" class="TabCtl (严格)"(error in=w163, "Value"=T18."模拟丢失" ("动作输出")) -> (error out=w159:errorcluster)  [unwired: 1 in, 1 out]
      n144 = property on="BTR0" class="DigNum (严格)"("DisabledEnum"=w193) -> ()  [unwired: 2 in, 2 out]
      n145 = property on="BTR1" class="DigNum (严格)"("DisabledEnum"=w193) -> ()  [unwired: 2 in, 2 out]
      n146 = global write "GlobalVariable.vi" "Success"(w164) -> ()
      n147 = global write "GlobalVariable.vi" "Exit"(w164) -> ()
      n148 = global write "GlobalVariable.vi" "计数清零"(FALSE) -> ()
      n149 = property on="OpenDevice" class="Bool (严格)"("BoolText.Text"="打开设备" ("布尔文本.文本")) -> ()  [unwired: 2 in, 2 out]
      n150 = global write "GlobalVariable.vi" "列累计"(string[] [] ("列累计")) -> ()
      n151 = Create User Event(user event datatype="TREvent", error in=w159) -> (user event=w190:refnum<user-event>, error out=w192:errorcluster)
      n152 = Create User Event(user event datatype="Log", error in=w159) -> (user event=w171:refnum<user-event>, error out=w175:errorcluster)
      n153 = flat-sequence {
        tunnel: w171 -> [w196]
        tunnel: [w196] -> w161
        tunnel: w161 -> [_]
        tunnel: [w197] -> w160
        frame #0 {
          "LogEvent" <- w196
        }
        frame #1 {
          n154 = control-ref of="LogEvent"() -> (w197:refnum<vi>)
        }
      }
      n155 = register-events(error in=w192, w190) -> (reference out=w174:refnum<event-registration>, error out=w170:errorcluster)  [unwired: 1 in]
      n156 = register-events(error in=w175, w171) -> (reference out=w173:refnum<event-registration>, error out=w169:errorcluster)  [unwired: 1 in]
      n157 = property on="界面标识" class="Str"("Value"="发送界面" ("界面标识")) -> (error out=w166:errorcluster)  [unwired: 2 in, 1 out]
      n158 = property on="多列列表框" class="MCListbox (严格)"("ItemNames"=string[][] [] ("项名")) -> ()  [unwired: 2 in, 2 out]
      n159 = property on="界面标识" class="Str"(error in=w166, "Text.TextColor"=u32 16711680, "Text.FontBold"=TRUE, "Text.BGColor"=u32 16777088, "Text.FontItalic"=FALSE) -> ()  [unwired: 1 in, 2 out]
      n160 = Bundle("事件注册引用句柄"=w174, "事件注册引用句柄"=w173) -> (w172:T32)  [unwired: 1 in]
      n161 = Merge Errors(w170, w169) -> (w168:errorcluster)
      n162 = control-ref of="消息"() -> (w165:refnum<vi>)
    }
  }
  n163 = while {
    tunnel: w7 -> [w202]
    tunnel: w6 -> [w201]
    tunnel: w5 -> [w200]
    tunnel: [w198] -> w4
    i -> [w204]
    stop <- w207 stop-if-true
    # "任意ID周期发送"
    n164 = local read "CANStartup"() -> (w206:bool)
    n165 = case shown="无错误" w202 {
      selector: w202 -> [w208 w291]
      tunnel: w206 -> [w215 _]
      tunnel: [w214 TRUE ("Exit")] -> w205
      tunnel: [w209 w291] -> w198
      tunnel: w204 -> [w213 _]
      tunnel: w201 -> [w212 _]
      tunnel: w200 -> [w211 _]
      tunnel: "Transmit" -> [w210 _]
      frame No Error {
        n166 = case shown="真" w215 {
          tunnel: [w218 w227] -> w214
          tunnel: w213 -> [_ w226]
          tunnel: w212 -> [_ w224]
          tunnel: w211 -> [_ w221]
          tunnel: w210 -> [_ w220]
          tunnel: [w216 w219] -> w209
          tunnel: w208 -> [w216 _]
          frame False {
            # "这个延时必须要，不然程序卡在此处"
            n167 = Wait (ms)(milliseconds to wait=u32 2 ("等待时间（毫秒）")) -> ()  [unwired: 1 out]
            n168 = global read "GlobalVariable.vi" "Exit"() -> (w218:bool)
          }
          frame True {
            n169 = flat-sequence {
              tunnel: [w250] -> w233
              tunnel: [w249] -> w232
              tunnel: [w248] -> w231
              tunnel: [w247] -> w230
              tunnel: [w246] -> w229
              tunnel: ["周期"] -> w228
              tunnel: [w246] -> w227
              tunnel: w226 -> [w244]
              tunnel: [w239] -> w225
              tunnel: w224 -> [w239]
              tunnel: [w236] -> w223
              tunnel: [w235] -> w222
              tunnel: w221 -> [w235]
              tunnel: w220 -> [w234]
              tunnel: w233 -> [w273]
              tunnel: w232 -> [w272]
              tunnel: w231 -> [w271]
              tunnel: w230 -> [w270]
              tunnel: w229 -> [w268]
              tunnel: w228 -> [w269]
              tunnel: w225 -> [w267]
              tunnel: w223 -> [w266]
              tunnel: w222 -> [w265]
              tunnel: [w264] -> w219
              frame #0 {
                n170 = local read "VCI_CAN_OBJ_T"() -> (w240:T9)
                n171 = To Unsigned Byte Integer(number=w244) -> (unsigned 8bit integer=w243:u8)
                n172 = call "ArrayConstant.vi"() -> ("VCI_CAN_OBJ_RN"=w245:T7)
                n173 = Number To Decimal String(number=w243) -> (decimal integer string=w237:string)  [unwired: 1 in]
                n174 = for {
                  N: 1 -> [_]
                  shift-right: [w258] -> w247
                  shift-left: w245 -> [w259]
                  tunnel: w234 -> [w257]
                  tunnel: w240 -> [w256]
                  n175 = case shown="真" w257 {
                    tunnel: w259 -> [w260 w263]
                    tunnel: [w260 w262] -> w258
                    tunnel: w256 -> [_ w261]
                    frame False {
                    }
                    frame True {
                      n176 = Insert Into Array(array=w263, new element=w261) -> (w262:T7)  [unwired: 1 in]
                    }
                  }
                }
                n177 = local read "CAN 通道"() -> (w253:u32)
                n178 = local read "设备类型"() -> (w255:u32)
                n179 = local read "索引"() -> (w254:u32)
                n180 = Concatenate Strings("任意ID发送失败！", w237) -> (w236:string)
                n181 = Array Size(array=w247) -> (size(s)=w252:i32)
                n182 = local read "VCI_CAN_OBJ_T"() -> (w248:T9)
                n183 = To Unsigned Long Integer(number=w252) -> (unsigned 32bit integer=w251:u32)
                n184 = dll-call lib="PTH1?abs E源码LV源码CAN\nCAN_ZLG3.7CANControlCAN.dll" fn="VCI_Transmit"("DeviceType"=w255, "DeviceInd"=w254, "CANInd"=w253, "pSend"=w247, "Len"=w252) -> ("return type"=w249:u32)  [unwired: 7 in, 3 out]
                n185 = global read "GlobalVariable.vi" "Exit"() -> (w246:bool)
                n186 = Greater Or Equal?(x=w249, y=w251) -> (x >= y?=w250:bool)
              }
              frame #1 {
                n187 = case shown="真" w273 {
                  tunnel: w271 -> [_ w288]
                  tunnel: w272 -> [_ w287]
                  tunnel: w270 -> [_ w285]
                  tunnel: w268 -> [_ _]
                  tunnel: w267 -> [_ w283]
                  tunnel: w266 -> [w277 _]
                  tunnel: w265 -> [w276 _]
                  tunnel: [w275 w282] -> w264
                  frame False {
                    n188 = Bundle By Name(cluster=T3 {"Event"="", "Value"=variant} ("Log"), "Event"="Error", "Value"=w277) -> (w280:T3)
                    n189 = Generate User Event(user event=w276, event data cluster=w280) -> (error out=w278:errorcluster)  [unwired: 2 in, 1 out]
                    n190 = call <vilib>:"Clear Errors.vi"("error in (no error)"=w278) -> ("error out"=w275:errorcluster)  [unwired: 6 in]
                  }
                  frame True {
                    n191 = Bundle(TRUE, "VCI_CAN_OBJ_T"=w288, "VCI_CAN_OBJ_RN"=w285, "return type"=w287) -> (w286:T33)  [unwired: 1 in]
                    n192 = Generate User Event(user event=w283, event data cluster=w286) -> (error out=w284:errorcluster)  [unwired: 2 in, 1 out]
                    n193 = call <vilib>:"Clear Errors.vi"("error in (no error)"=w284) -> ("error out"=w282:errorcluster)  [unwired: 6 in]
                  }
                }
                n194 = case shown="假" w268 {
                  tunnel: w269 -> [w274 _]
                  frame False {
                    n195 = Wait (ms)(milliseconds to wait=w274) -> ()  [unwired: 1 out]
                  }
                  frame True {
                  }
                }
              }
            }
          }
        }
      }
      frame Error {
      }
    }
    n196 = global read "GlobalVariable.vi" "Exit"() -> (w203:bool)
    n197 = Compound Arithmetic op=OR(w198, w205, w203) -> (w207:bool)
  }
  n198 = while {
    tunnel: w34 -> [w301]
    tunnel: [w300] -> w33
    tunnel: w8 -> [w299]
    tunnel: w3 -> [w298]
    tunnel: w10 -> [w297]
    shift-right: [w295] -> _
    shift-left: "" -> [w296]
    tunnel: w9 -> [w292]
    stop <- w294 stop-if-true
    n199 = event shown="[1] <事件注册引用句柄.TREvent>: 用户事件" {
      selector: w301 -> [_ _ _]
      dyn-events: [_ _ _] -> w300
      timeout: 5 -> [_ _ _]
      tunnel: [FALSE _ _] -> w303
      tunnel: w299 -> [_ w311 _]
      tunnel: w298 -> [_ w310 _]
      tunnel: w297 -> [_ _ w385]
      tunnel: w296 -> [w304 w309 w384]
      tunnel: [w304 w309 w383] -> w295
      tunnel: w292 -> [_ w308 _]
      event Timeout {
        n200 = event-data() -> ()  [unwired: 1 in, 1 out]
      }
      event User Event {
        n201 = event-data() -> ("Tx_Or_Rx"=w318:bool, "VCI_CAN_OBJ_N"=w312:T7, "Num"=w315:u32)  [unwired: 1 in, 1 out]
        n202 = control-ref of="多列列表框"() -> (w320:refnum<vi>)
        n203 = Greater Or Equal?(x=w315, y=u32 1) -> (x >= y?=w316:bool)
        n204 = Not(x=w318) -> (.not. x?=w317:bool)
        n205 = And(x=w317, y=w316) -> (x .and. y?=w313:bool)
        n206 = global read "GlobalVariable.vi" "计数清零"() -> (w306:bool)
        n207 = case shown="真" w313 {
          tunnel: w312 -> [_ w336]
          tunnel: w311 -> [_ w335]
          tunnel: w310 -> [_ w334]
          tunnel: w308 -> [_ w333]
          frame False {
          }
          frame True {
            n208 = Array Size(array=w336) -> (size(s)=w337:i32)
            n209 = for {
              N: w337 -> [_]
              tunnel: w336 -> [w341] mode=indexing
              tunnel: w335 -> [w340]
              tunnel: w334 -> [w339]
              tunnel: w333 -> [w338]
              n210 = call "ReceiveStringCheck.vi"("VCI_CAN_OBJ_R"=w341) -> ("约定ID"=w342:string)
              n211 = case shown="\"2AF\"" w342 {
                tunnel: w341 -> [_ w344 w353 w356 w362 w367 w369 w375 w377 w380]
                tunnel: w340 -> [_ _ _ _ w360 w366 _ w373 _ _]
                tunnel: w339 -> [_ _ _ _ w359 w365 _ w372 _ _]
                tunnel: w338 -> [_ w343 w352 w355 w358 w363 w368 w371 w376 w379]
                frame Default {
                }
                frame "2AF" {
                  n212 = call "TimeStrDismantle.vi"("LogEvent"=w343, "VCI_CAN_OBJ_R"=w344) -> ("TimeCluster"=w351:T34)
                  n213 = Unbundle By Name(w351) -> ("秒"=w350:i32, "分"=w349:i32, "时"=w348:i32, "日"=w347:i32, "月"=w346:i32, "年"=w345:i32)
                  n214 = local write "秒"(w350) -> ()
                  n215 = local write "分"(w349) -> ()
                  n216 = local write "时"(w348) -> ()
                  n217 = local write "日"(w347) -> ()
                  n218 = local write "月"(w346) -> ()
                  n219 = local write "年"(w345) -> ()
                }
                frame "3E1" {
                  n220 = call "GPS_StrDismantle_3E1.vi"("LogEvent"=w352, "VCI_CAN_OBJ_R"=w353) -> ("GPS位置信息1"=w354:T11)
                  n221 = property on="GPS位置信息1" class="Clust (严格)"("Value"=w354) -> ()  [unwired: 2 in, 2 out]
                }
                frame "3E2" {
                  n222 = call "GPS_StrDismantle_3E2.vi"("LogEvent"=w355, "VCI_CAN_OBJ_R"=w356) -> ("GPS位置信息2"=w357:T11)
                  n223 = property on="GPS位置信息2" class="Clust (严格)"("Value"=w357) -> ()  [unwired: 2 in, 2 out]
                }
                frame "2A1" {
                  n224 = call "MMI_BCM_StrDismantle.vi"("LogEvent"=w358, "VCI_CAN_OBJ_R"=w362) -> ("BCM_CmdCluster"=w361:T35)
                  "BCM" <- w361
                  n225 = call "MMI_BCM_2A1_Action.vi"("Input2"=w359, "Input1"=w360, "BCM"=w361) -> ()  [unwired: 8 in, 1 out]
                }
                frame "2A5" {
                  n226 = call "MMI_AC_StrDismantle.vi"("LogEvent"=w363, "VCI_CAN_OBJ_R"=w367) -> ("MMI_AC_CmdCluster"=w364:T36)
                  "AC空调" <- w364
                  n227 = call "MMI_AC_2A5_Action.vi"("Input2"=w365, "Input1"=w366, "AC空调"=w364) -> ()  [unwired: 8 in, 1 out]
                }
                frame "2A4" {
                  n228 = call "MMI_ButtonSkin_StrDismantle.vi"("LogEvent"=w368, "VCI_CAN_OBJ_R"=w369) -> ("MMI_ButtonSkin_CmdCluster"=→"Skin":T14)
                }
                frame "2A7" {
                  n229 = call "MMI_PEPS_StrDismantle.vi"("LogEvent"=w371, "VCI_CAN_OBJ_R"=w375) -> ("MMI_PEPS_CmdCluster"=w374:T37)
                  "PEPS" <- w374
                  n230 = call "MMI_PEPS_2A7_Action.vi"("Input2"=w372, "Input1"=w373, "PEPS"=w374) -> ()  [unwired: 8 in, 1 out]
                }
                frame "2D0" {
                  n231 = call "MMI_Intelligent_StrDismantle.vi"("LogEvent"=w376, "VCI_CAN_OBJ_R"=w377) -> ("MMI_ItelligentCmdCluster"=→"智能信号管理":T38)
                }
                frame "2A8" {
                  n232 = call "MMI_PAS_StrDismantle.vi"("LogEvent"=w379, "VCI_CAN_OBJ_R"=w380) -> ("MMI_PAS_CmdCluster"=→"PAS_FCS":T17)
                }
              }
            }
          }
        }
        n233 = case shown="真" "刷新" {
          tunnel: w320 -> [w321 w330]
          tunnel: [w326 w332] -> w319
          tunnel: w318 -> [w325 w331]
          tunnel: w315 -> [w324 w329]
          tunnel: w312 -> [w323 w328]
          tunnel: w306 -> [w322 w327]
          frame False {
            n234 = call "MulticolumnView.vi"("CountClear"=w322, "VCI_CAN_OBJ_N"=w323, "Num"=w324, "MCListbox引用句柄"=w321, "Tx_Or_Rx"=w325) -> ("MCListbox输出"=w326:refnum<vi>)  [unwired: 6 in]
          }
          frame True {
            n235 = call "MulticolumnViewSX.vi"("CountClear"=w327, "VCI_CAN_OBJ_N"=w328, "Num"=w329, "MCListbox引用句柄"=w330, "Tx_Or_Rx"=w331) -> ("MCListbox输出"=w332:refnum<vi>)  [unwired: 6 in]
          }
        }
        n236 = flat-sequence {
          tunnel: w319 -> [_]
          frame #0 {
            n237 = global write "GlobalVariable.vi" "计数清零"(FALSE) -> ()
          }
        }
      }
      event User Event {
        n238 = event-data() -> ("Event"=w389:string, "Value"=w388:variant)  [unwired: 1 in]
        n239 = Variant To Data(type="", Variant=w388) -> (data=w386:string)  [unwired: 1 in, 1 out]
        n240 = case shown="\"Error\"" w389 {
          tunnel: w386 -> [_ w395]
          tunnel: w385 -> [_ w394]
          tunnel: w384 -> [w390 w396]
          tunnel: [w390 w391] -> w383
          frame "假", Default {
          }
          frame "Error" {
            n241 = Concatenate Strings(w396, w395, "\n") -> (w391:string)
            n242 = String Length(string=w391) -> (length=w392:i32)
            n243 = property class="Str"(reference=w394, "Text.Text"=w391, "Text.Scroll Position"=w392) -> ()  [unwired: 1 in, 2 out]
          }
        }
      }
    }
    n244 = global read "GlobalVariable.vi" "Exit"() -> (w293:bool)
    n245 = Compound Arithmetic op=OR(w293, w303) -> (w294:bool)
  }
  n246 = while {
    tunnel: w10 -> [w400]
    tunnel: w8 -> [w399]
    tunnel: w3 -> [w398]
    tunnel: [w397] -> w1
    stop <- w402 stop-if-true
    n247 = event shown="[1] \"Clear Buffer\", \"刷新\": 值改变" {
      selector: _ -> [_ _ _ _ _ _ _ _ _ _ _ _ _ _]
      dyn-events: _ -> [_ _ _ _ _ _ _ _ _ _ _ _ _ _]
      timeout: 10 -> [_ _ _ _ _ _ _ _ _ _ _ _ _ _]
      tunnel: [w403 _ _ _ _ _ _ _ _ _ _ _ w606 _] -> w402
      tunnel: w400 -> [_ w415 _ _ _ _ _ _ _ _ w599 _ _ _]
      tunnel: w399 -> [_ _ _ _ _ _ _ _ _ _ _ w604 _ w616]
      tunnel: w398 -> [_ _ _ _ _ _ _ _ _ _ w601 _ _ _]
      tunnel: [_ _ _ _ _ _ _ _ _ _ w599 _ _ _] -> w397
      event "退出": Value Change {
        n248 = event-data() -> ()  [unwired: 1 in, 1 out]
        n249 = Two Button Dialog(message="程序正在运行确定退出？" ("消息")) -> (T button?=w405:bool)  [unwired: 2 in]
        n250 = case shown="真" w405 {
          tunnel: [_ w406] -> w403
          frame False {
          }
          frame True {
            n251 = stacked-sequence {
              tunnel: [_ _ w412] -> w406
              frame #0 {
                n252 = local read "设备类型"() -> (w408:u32)
                n253 = local write "CANStartup"(FALSE) -> ()
                n254 = dll-call lib="PTH1?abs E源码LV源码CAN\nCAN_ZLG3.7CANControlCAN.dll" fn="VCI_CloseDevice"("DeviceType"=w408, "DeviceInd"=0) -> ()  [unwired: 5 in, 3 out]
              }
              frame #1 {
                # "这个延时必须要"
                n255 = property on="设备类型" class="Ring (严格)"("DisabledEnum"=T39."Enabled" ("禁用")) -> ()  [unwired: 2 in, 2 out]
                n256 = Wait (ms)(milliseconds to wait=u32 500 ("等待时间（毫秒）")) -> ()  [unwired: 1 out]
              }
              frame #2 {
                w412 = TRUE
                n257 = global write "GlobalVariable.vi" "Exit"(w412) -> ()
              }
            }
          }
        }
      }
      event "Clear Buffer", "刷新": Value Change {
        n258 = event-data() -> ()  [unwired: 1 in, 1 out]
        n259 = local read "DevOpen"() -> (w418:bool)
        n260 = case shown="真" w418 {
          frame False {
          }
          frame True {
            n261 = local read "CAN 通道"() -> (w419:u32)
            n262 = local read "设备类型"() -> (w421:u32)
            n263 = local read "索引"() -> (w420:u32)
            n264 = dll-call lib="PTH1?abs E源码LV源码CAN\nCAN_ZLG3.7CANControlCAN.dll" fn="VCI_ClearBuffer"("DeviceType"=w421, "DeviceInd"=w420, "CANInd"=w419) -> ()  [unwired: 6 in, 3 out]
          }
        }
        n265 = global write "GlobalVariable.vi" "列累计"(string[] [] ("列累计")) -> ()
        n266 = property class="Str"(reference=w415, "Text.Text"="") -> ()  [unwired: 1 in, 2 out]
        n267 = global write "GlobalVariable.vi" "计数清零"(TRUE) -> ()
        n268 = property on="多列列表框" class="MCListbox (严格)"("ItemNames"=string[][] [] ("项名")) -> ()  [unwired: 2 in, 2 out]
      }
      event Menu Selection (User) {
        n269 = event-data() -> ("ItemTag"=w422:string)  [unwired: 1 in]
        n270 = case shown="\"Received\", 默认" w422 {
          frame "Received", Default {
            n271 = property on="前面板显示" class="TabCtl (严格)"("Value"=enum32{"接收", "发送", "帮助"}."接收" ("前面板显示")) -> ()  [unwired: 2 in, 2 out]
            n272 = property on="界面标识" class="Str"("Value"="显示界面" ("界面标识")) -> ()  [unwired: 2 in, 2 out]
          }
          frame "Transmited" {
            n273 = property on="界面标识" class="Str"("Value"="发送界面" ("界面标识")) -> ()  [unwired: 2 in, 2 out]
            n274 = property on="前面板显示" class="TabCtl (严格)"("Value"=enum32{"接收", "发送", "帮助"}."发送" ("前面板显示")) -> ()  [unwired: 2 in, 2 out]
          }
          frame "Help" {
            n275 = property on="前面板显示" class="TabCtl (严格)"("Value"=enum32{"接收", "发送", "帮助"}."帮助" ("前面板显示")) -> ()  [unwired: 2 in, 2 out]
            n276 = property on="界面标识" class="Str"("Value"="帮助界面" ("界面标识")) -> ()  [unwired: 2 in, 2 out]
          }
          frame "About" {
            n277 = call "About.vi"() -> ()  [unwired: 12 in]
          }
        }
      }
      event "GetStatus": Value Change {
        n278 = event-data() -> ()  [unwired: 1 in, 1 out]
        n279 = local read "CAN 通道"() -> (w431:u32)
        n280 = local read "设备类型"() -> (w429:u32)
        n281 = local read "索引"() -> (w430:u32)
        n282 = dll-call lib="PTH1?abs E源码LV源码CAN\nCAN_ZLG3.7CANControlCAN.dll" fn="VCI_ReadCANStatus"("DeviceType"=w429, "DeviceInd"=w430, "CANInd"=w431) -> ("VCI_CAN_STATUS"=w432:T5)  [unwired: 6 in, 4 out]
        "VCI_CAN_STATUS" <- w432
        n283 = call "status.vi"("VCI_CAN_STATUS"=w432) -> ()  [unwired: 1 in]
      }
      event "GetErrorInfo": Value Change {
        n284 = event-data() -> ()  [unwired: 1 in, 1 out]
        n285 = local read "CAN 通道"() -> (w435:u32)
        n286 = local read "设备类型"() -> (w433:u32)
        n287 = local read "索引"() -> (w434:u32)
        n288 = dll-call lib="PTH1?abs E源码LV源码CAN\nCAN_ZLG3.7CANControlCAN.dll" fn="VCI_ReadErrInfo"("DeviceType"=w433, "DeviceInd"=w434, "CANInd"=w435) -> ("VCI_ERR_INFO"=w436:T6)  [unwired: 6 in, 4 out]
        "VCI_ERR_INFO" <- w436
        n289 = call "errinfo.vi"("VCI_ERR_INFO"=w436) -> ()  [unwired: 1 in]
      }
      event "Baud": Value Change {
        n290 = event-data() -> ("NewVal"=w437:u32)  [unwired: 1 in]
        n291 = case shown="15, 默认" w437 {
          frame 0 {
            n292 = local write "BTR0"(u8 191 ("BTR0")) -> ()
            n293 = local write "BTR1"(u8 255 ("BTR1")) -> ()
          }
          frame 1 {
            n294 = local write "BTR0"(49) -> ()
            n295 = local write "BTR1"(28) -> ()
          }
          frame 2 {
            n296 = local write "BTR1"(28) -> ()
            n297 = local write "BTR0"(24) -> ()
          }
          frame 3 {
            n298 = local write "BTR0"(135) -> ()
            n299 = local write "BTR1"(255) -> ()
          }
          frame 4 {
            n300 = local write "BTR0"(9) -> ()
            n301 = local write "BTR1"(28) -> ()
          }
          frame 5 {
            n302 = local write "BTR0"(131) -> ()
            n303 = local write "BTR1"(255) -> ()
          }
          frame 6 {
            n304 = local write "BTR0"(4) -> ()
            n305 = local write "BTR1"(28) -> ()
          }
          frame 7 {
            n306 = local write "BTR0"(3) -> ()
            n307 = local write "BTR1"(28) -> ()
          }
          frame 8 {
            n308 = local write "BTR0"(129) -> ()
            n309 = local write "BTR1"(250) -> ()
          }
          frame 9 {
            n310 = local write "BTR0"(1) -> ()
            n311 = local write "BTR1"(28) -> ()
          }
          frame 10 {
            n312 = local write "BTR0"(128) -> ()
            n313 = local write "BTR1"(250) -> ()
          }
          frame 11 {
            n314 = local write "BTR0"(0) -> ()
            n315 = local write "BTR1"(28) -> ()
          }
          frame 12 {
            n316 = local write "BTR0"(128) -> ()
            n317 = local write "BTR1"(182) -> ()
          }
          frame 13 {
            n318 = local write "BTR0"(0) -> ()
            n319 = local write "BTR1"(22) -> ()
          }
          frame 14 {
            n320 = local write "BTR1"(20) -> ()
            n321 = local write "BTR0"(0) -> ()
          }
          frame 15, Default {
            n322 = local write "BTR0"(1) -> ()
            n323 = local write "BTR1"(1) -> ()
          }
        }
      }
      event "滤波": Value Change {
        n324 = event-data() -> ("NewVal"=w470:bool)  [unwired: 1 in]
        n325 = stacked-sequence {
          seq-local: [w472 _] -> [_ w477]
          seq-local: [w471 _] -> [_ w476]
          tunnel: w470 -> [w472 _]
          frame #0 {
            n326 = Number To Hexadecimal String(2:"滤波ID") -> (0:w471:string)  [unwired: 1 in]
            n327 = call "Filter.vi"("滤波"=w472, "ID(Hex 高位有效)"=w471) -> ("屏蔽码"=w473:u32, "验收码"=w474:u32)  [unwired: 8 in]
            n328 = property on="屏蔽码" class="DigNum (严格)"("Value"=w473) -> ()  [unwired: 2 in, 2 out]
            n329 = property on="验收码" class="DigNum (严格)"("Value"=w474) -> ()  [unwired: 2 in, 2 out]
          }
          frame #1 {
            n330 = case shown="真" w477 {
              tunnel: w476 -> [w478 w499]
              frame False {
                n331 = stacked-sequence {
                  tunnel: w478 -> [_ w486 _]
                  frame #0 {
                    n332 = local read "设备类型"() -> (w482:u32)
                    n333 = local read "索引"() -> (w481:u32)
                    n334 = dll-call lib="PTH1?abs E源码LV源码CAN\nCAN_ZLG3.7CANControlCAN.dll" fn="VCI_CloseDevice"("DeviceType"=w482, "DeviceInd"=w481) -> (error out=w480:errorcluster)  [unwired: 5 in, 2 out]
                    n335 = call "时间延迟9"("error in (no error)"=w480, "Delay Time (s)"=0.5) -> ()  [unwired: 9 in, 1 out]
                  }
                  frame #1 {
                    n336 = disable-structure shown="启用" {
                      disable-tunnel: w486 -> [w491 _]
                      disable-tunnel: [w488 w495] -> w485
                      disable-tunnel: [w487 w495] -> w484
                      frame Disabled {
                        n337 = local read "设备类型"() -> (w494:u32)
                        n338 = local read "Baud"() -> (w490:u32)
                        n339 = call "OpenDevice.vi"("设备类型"=w494) -> ("错误输出"=w489:errorcluster, "Result"=w488:bool, "DevType"=w493:u32)  [unwired: 8 in]
                        n340 = call "InitDevice.vi"("滤波"=FALSE, "错误输入（无错误）"=w489, "Baud"=w490, "ID(Hex 高位有效)"=w491, "设备类型"=w493) -> ("Result"=w487:bool)  [unwired: 4 in, 2 out]
                      }
                      frame Enabled {
                        w495 = FALSE
                        n341 = local write "OpenDevice"(w495) -> ()
                      }
                    }
                    n342 = property on="OpenDevice" class="Bool (严格)"("BoolText.Text"="打开设备" ("布尔文本.文本")) -> ()  [unwired: 2 in, 2 out]
                    n343 = local write "DevOpen"(w485) -> ()
                    n344 = local write "CANStartup"(w484) -> ()
                  }
                  frame #2 {
                    w496 = 0
                    w498 = 0
                    w497 = 0
                    n345 = property on="验收码" class="DigNum (严格)"("DisabledEnum"=w497) -> ()  [unwired: 2 in, 2 out]
                    n346 = property on="屏蔽码" class="DigNum (严格)"("DisabledEnum"=w497) -> ()  [unwired: 2 in, 2 out]
                    n347 = property on="Baud" class="Ring (严格)"("DisabledEnum"=w497) -> ()  [unwired: 2 in, 2 out]
                    n348 = property on="BTR0" class="DigNum (严格)"("DisabledEnum"=w497) -> ()  [unwired: 2 in, 2 out]
                    n349 = property on="CAN 通道" class="Ring (严格)"("DisabledEnum"=w497) -> ()  [unwired: 2 in, 2 out]
                    n350 = property on="设备类型" class="Ring (严格)"("DisabledEnum"=w496) -> ()  [unwired: 2 in, 2 out]
                    n351 = property on="滤波ID" class="DigNum (严格)"("DisabledEnum"=w496) -> ()  [unwired: 2 in, 2 out]
                    n352 = property on="OpenDevice" class="Bool (严格)"("DisabledEnum"=w496) -> ()  [unwired: 2 in, 2 out]
                    n353 = property on="ResetCAN" class="Bool (严格)"("DisabledEnum"=w496) -> ()  [unwired: 2 in, 2 out]
                    n354 = property on="StartCAN" class="Bool (严格)"("DisabledEnum"=w496) -> ()  [unwired: 2 in, 2 out]
                    n355 = property on="滤波方式" class="Ring (严格)"("DisabledEnum"=w498) -> ()  [unwired: 2 in, 2 out]
                    n356 = property on="模式" class="Ring (严格)"("DisabledEnum"=w498) -> ()  [unwired: 2 in, 2 out]
                    n357 = property on="BTR1" class="DigNum (严格)"("DisabledEnum"=w498) -> ()  [unwired: 2 in, 2 out]
                    n358 = property on="索引" class="Ring (严格)"("DisabledEnum"=w498) -> ()  [unwired: 2 in, 2 out]
                  }
                }
              }
              frame True {
                n359 = stacked-sequence {
                  tunnel: w499 -> [_ w508 _]
                  frame #0 {
                    n360 = local read "设备类型"() -> (w503:u32)
                    n361 = local read "索引"() -> (w502:u32)
                    n362 = dll-call lib="PTH1?abs E源码LV源码CAN\nCAN_ZLG3.7CANControlCAN.dll" fn="VCI_CloseDevice"("DeviceType"=w503, "DeviceInd"=w502) -> (error out=w501:errorcluster)  [unwired: 5 in, 2 out]
                    n363 = call "时间延迟8"("error in (no error)"=w501, "Delay Time (s)"=0.5) -> ()  [unwired: 9 in, 1 out]
                  }
                  frame #1 {
                    n364 = local read "设备类型"() -> (w511:u32)
                    n365 = local read "Baud"() -> (w507:u32)
                    n366 = call "OpenDevice.vi"("设备类型"=w511) -> ("错误输出"=w506:errorcluster, "Result"=w505:bool, "DevType"=w510:u32)  [unwired: 8 in]
                    n367 = local write "DevOpen"(w505) -> ()
                    n368 = call "InitDevice.vi"("滤波"=TRUE, "错误输入（无错误）"=w506, "Baud"=w507, "ID(Hex 高位有效)"=w508, "设备类型"=w510) -> ("Result"=w504:bool)  [unwired: 4 in, 2 out]
                    n369 = local write "CANStartup"(w504) -> ()
                  }
                  frame #2 {
                    w512 = 2
                    w513 = 2
                    w514 = 2
                    n370 = property on="验收码" class="DigNum (严格)"("DisabledEnum"=w514) -> ()  [unwired: 2 in, 2 out]
                    n371 = property on="屏蔽码" class="DigNum (严格)"("DisabledEnum"=w514) -> ()  [unwired: 2 in, 2 out]
                    n372 = property on="Baud" class="Ring (严格)"("DisabledEnum"=w514) -> ()  [unwired: 2 in, 2 out]
                    n373 = property on="BTR0" class="DigNum (严格)"("DisabledEnum"=w514) -> ()  [unwired: 2 in, 2 out]
                    n374 = property on="CAN 通道" class="Ring (严格)"("DisabledEnum"=w514) -> ()  [unwired: 2 in, 2 out]
                    n375 = property on="ResetCAN" class="Bool (严格)"("DisabledEnum"=w512) -> ()  [unwired: 2 in, 2 out]
                    n376 = property on="StartCAN" class="Bool (严格)"("DisabledEnum"=w512) -> ()  [unwired: 2 in, 2 out]
                    n377 = property on="设备类型" class="Ring (严格)"("DisabledEnum"=w512) -> ()  [unwired: 2 in, 2 out]
                    n378 = property on="滤波ID" class="DigNum (严格)"("DisabledEnum"=w512) -> ()  [unwired: 2 in, 2 out]
                    n379 = property on="滤波方式" class="Ring (严格)"("DisabledEnum"=w513) -> ()  [unwired: 2 in, 2 out]
                    n380 = property on="模式" class="Ring (严格)"("DisabledEnum"=w513) -> ()  [unwired: 2 in, 2 out]
                    n381 = property on="BTR1" class="DigNum (严格)"("DisabledEnum"=w513) -> ()  [unwired: 2 in, 2 out]
                    n382 = property on="索引" class="Ring (严格)"("DisabledEnum"=w513) -> ()  [unwired: 2 in, 2 out]
                    n383 = property on="OpenDevice" class="Bool (严格)"("DisabledEnum"=w513) -> ()  [unwired: 2 in, 2 out]
                  }
                }
              }
            }
          }
        }
      }
      event "OpenDevice": Value Change {
        n384 = event-data() -> ()  [unwired: 1 in, 1 out]
        n385 = case shown="假" "DevOpen" {
          frame False {
            n386 = local read "索引"() -> (w516:u32)
            n387 = dll-call lib="PTH1?abs E源码LV源码CAN\nCAN_ZLG3.7CANControlCAN.dll" fn="VCI_OpenDevice" label="OpenDevice"("DevType"="设备类型", "DevIndex"=w516, "Reserved"=u32 0) -> ("返回类型"=w521:u32)  [unwired: 6 in, 2 out]
            n388 = Equal?(x=w521, y=u32 1) -> (x = y?=w519:bool)
            n389 = case shown="真" w519 {
              selector: w519 -> [w522 _]
              frame False {
                n390 = global write "GlobalVariable.vi" "Success"(w522) -> ()
                n391 = call "显示对话框信息"() -> ()  [unwired: 3 in, 9 out]
              }
              frame True {
                n392 = stacked-sequence {
                  frame #0 {
                    n393 = property on="设备类型" class="Ring (严格)"() -> (error out=w530:errorcluster, "Value"=w529:u32)  [unwired: 2 in, 1 out]
                    n394 = local read "索引"() -> (w527:u32)
                    n395 = local read "CAN 通道"() -> (w526:u32)
                    n396 = local read "VCI_INIT_CONFIG"() -> (w528:T8)
                    n397 = dll-call lib="PTH1?abs E源码LV源码CAN\nCAN_ZLG3.7CANControlCAN.dll" fn="VCI_InitCAN"(error in=w530, "DeviceType"=w529, "DeviceInd"=w527, "CANInd"=w526, "pInitConfig"=w528) -> ("返回类型"=w525:u32)  [unwired: 6 in, 2 out]
                    n398 = Equal?(x=w525, y=u32 1) -> (x = y?=w523:bool)
                    n399 = case shown="假" w523 {
                      frame False {
                        n400 = call "显示对话框信息2"() -> ()  [unwired: 3 in, 9 out]
                      }
                      frame True {
                      }
                    }
                    n401 = global write "GlobalVariable.vi" "Success"(w523) -> ()
                  }
                  frame #1 {
                    n402 = global read "GlobalVariable.vi" "Success"() -> (w531:bool)
                    n403 = case shown="假" w531 {
                      frame False {
                        n404 = local read "设备类型"() -> (w533:u32)
                        n405 = local read "索引"() -> (w532:u32)
                        n406 = call "显示对话框信息3"() -> ()  [unwired: 3 in, 9 out]
                        n407 = dll-call lib="PTH1?abs E源码LV源码CAN\nCAN_ZLG3.7CANControlCAN.dll" fn="VCI_CloseDevice"("DeviceType"=w533, "DeviceInd"=w532) -> ()  [unwired: 5 in, 3 out]
                      }
                      frame True {
                        w534 = 2
                        w535 = 2
                        n408 = property on="设备类型" class="Ring (严格)"("DisabledEnum"=w535) -> ()  [unwired: 2 in, 2 out]
                        n409 = property on="验收码" class="DigNum (严格)"("DisabledEnum"=w535) -> ()  [unwired: 2 in, 2 out]
                        n410 = property on="屏蔽码" class="DigNum (严格)"("DisabledEnum"=w535) -> ()  [unwired: 2 in, 2 out]
                        n411 = property on="滤波方式" class="Ring (严格)"("DisabledEnum"=w535) -> ()  [unwired: 2 in, 2 out]
                        n412 = local write "DevOpen"(TRUE) -> ()
                        n413 = property on="OpenDevice" class="Bool (严格)"("BoolText.Text"="关闭设备") -> ()  [unwired: 2 in, 2 out]
                        n414 = property on="Baud" class="Ring (严格)"("DisabledEnum"=w534) -> ()  [unwired: 2 in, 2 out]
                        n415 = property on="BTR0" class="DigNum (严格)"("DisabledEnum"=w534) -> ()  [unwired: 2 in, 2 out]
                        n416 = property on="BTR1" class="DigNum (严格)"("DisabledEnum"=w534) -> ()  [unwired: 2 in, 2 out]
                        n417 = property on="模式" class="Ring (严格)"("DisabledEnum"=w534) -> ()  [unwired: 2 in, 2 out]
                      }
                    }
                  }
                }
              }
            }
          }
          frame True {
            n418 = stacked-sequence {
              frame #0 {
                n419 = local read "设备类型"() -> (w542:u32)
                n420 = local read "索引"() -> (w541:u32)
                n421 = dll-call lib="PTH1?abs E源码LV源码CAN\nCAN_ZLG3.7CANControlCAN.dll" fn="VCI_CloseDevice"("DeviceType"=w542, "DeviceInd"=w541) -> ("返回类型"=w540:u32)  [unwired: 5 in, 2 out]
                n422 = Equal?(x=w540, y=u32 1) -> (x = y?=w538:bool)
                n423 = case shown="真" w538 {
                  frame False {
                  }
                  frame True {
                    w543 = 0
                    w544 = 0
                    w546 = FALSE
                    n424 = property on="设备类型" class="Ring (严格)"("DisabledEnum"=w544) -> ()  [unwired: 2 in, 2 out]
                    n425 = property on="CAN 通道" class="Ring (严格)"("DisabledEnum"=w544) -> ()  [unwired: 2 in, 2 out]
                    n426 = property on="索引" class="Ring (严格)"("DisabledEnum"=w544) -> ()  [unwired: 2 in, 2 out]
                    n427 = property on="验收码" class="DigNum (严格)"("DisabledEnum"=w544) -> ()  [unwired: 2 in, 2 out]
                    n428 = property on="屏蔽码" class="DigNum (严格)"("DisabledEnum"=w544) -> ()  [unwired: 2 in, 2 out]
                    n429 = local write "DevOpen"(w546) -> ()
                    n430 = local write "CANStartup"(w546) -> ()
                    n431 = property on="OpenDevice" class="Bool (严格)"("BoolText.Text"="打开设备" ("布尔文本.文本")) -> ()  [unwired: 2 in, 2 out]
                    n432 = property on="BTR0" class="DigNum (严格)"("DisabledEnum"=w543) -> ()  [unwired: 2 in, 2 out]
                    n433 = property on="BTR1" class="DigNum (严格)"("DisabledEnum"=w543) -> ()  [unwired: 2 in, 2 out]
                    n434 = property on="模式" class="Ring (严格)"("DisabledEnum"=w543) -> ()  [unwired: 2 in, 2 out]
                    n435 = property on="Baud" class="Ring (严格)"("DisabledEnum"=w543) -> ()  [unwired: 2 in, 2 out]
                    n436 = property on="滤波方式" class="Ring (严格)"("DisabledEnum"=w543) -> ()  [unwired: 2 in, 2 out]
                  }
                }
              }
              frame #1 {
                w548 = 0
                w549 = 0
                n437 = property on="设备类型" class="Ring (严格)"("DisabledEnum"=w548) -> ()  [unwired: 2 in, 2 out]
                n438 = property on="CAN 通道" class="Ring (严格)"("DisabledEnum"=w548) -> ()  [unwired: 2 in, 2 out]
                n439 = property on="索引" class="Ring (严格)"("DisabledEnum"=w548) -> ()  [unwired: 2 in, 2 out]
                n440 = property on="验收码" class="DigNum (严格)"("DisabledEnum"=w548) -> ()  [unwired: 2 in, 2 out]
                n441 = property on="屏蔽码" class="DigNum (严格)"("DisabledEnum"=w548) -> ()  [unwired: 2 in, 2 out]
                n442 = property on="Baud" class="Ring (严格)"() -> ("Value"=w550:u32)  [unwired: 2 in, 2 out]
                n443 = Wait (ms)(milliseconds to wait=u32 500 ("等待时间（毫秒）")) -> ()  [unwired: 1 out]
                n444 = case shown="5" w550 {
                  frame 0 {
                    n445 = local write "BTR0"(u8 191 ("BTR0")) -> ()
                    n446 = local write "BTR1"(u8 255 ("BTR1")) -> ()
                  }
                  frame 1 {
                    n447 = local write "BTR0"(49) -> ()
                    n448 = local write "BTR1"(28) -> ()
                  }
                  frame 2 {
                    n449 = local write "BTR0"(24) -> ()
                    n450 = local write "BTR1"(28) -> ()
                  }
                  frame 3 {
                    n451 = local write "BTR0"(135) -> ()
                    n452 = local write "BTR1"(255) -> ()
                  }
                  frame 4 {
                    n453 = local write "BTR0"(9) -> ()
                    n454 = local write "BTR1"(28) -> ()
                  }
                  frame 5 {
                    n455 = local write "BTR0"(131) -> ()
                    n456 = local write "BTR1"(255) -> ()
                  }
                  frame 6 {
                    n457 = local write "BTR0"(4) -> ()
                    n458 = local write "BTR1"(28) -> ()
                  }
                  frame 7 {
                    n459 = local write "BTR0"(3) -> ()
                    n460 = local write "BTR1"(28) -> ()
                  }
                  frame 8 {
                    n461 = local write "BTR0"(129) -> ()
                    n462 = local write "BTR1"(250) -> ()
                  }
                  frame 9 {
                    n463 = local write "BTR0"(1) -> ()
                    n464 = local write "BTR1"(28) -> ()
                  }
                  frame 10 {
                    n465 = local write "BTR0"(128) -> ()
                    n466 = local write "BTR1"(250) -> ()
                  }
                  frame 11 {
                    n467 = local write "BTR0"(0) -> ()
                    n468 = local write "BTR1"(28) -> ()
                  }
                  frame 12 {
                    n469 = local write "BTR0"(128) -> ()
                    n470 = local write "BTR1"(182) -> ()
                  }
                  frame 13 {
                    n471 = local write "BTR0"(0) -> ()
                    n472 = local write "BTR1"(22) -> ()
                  }
                  frame 14 {
                    n473 = local write "BTR1"(20) -> ()
                    n474 = local write "BTR0"(0) -> ()
                  }
                  frame 15, Default {
                    n475 = local write "BTR0"(1) -> ()
                    n476 = local write "BTR1"(1) -> ()
                  }
                }
                n477 = property on="BTR0" class="DigNum (严格)"("DisabledEnum"=w549) -> ()  [unwired: 2 in, 2 out]
                n478 = property on="BTR1" class="DigNum (严格)"("DisabledEnum"=w549) -> ()  [unwired: 2 in, 2 out]
                n479 = property on="模式" class="Ring (严格)"("DisabledEnum"=w549) -> ()  [unwired: 2 in, 2 out]
                n480 = property on="Baud" class="Ring (严格)"("DisabledEnum"=w549) -> ()  [unwired: 2 in, 2 out]
              }
            }
          }
        }
      }
      event "StartCAN": Value Change {
        n481 = event-data() -> ()  [unwired: 1 in, 6 out]
        n482 = local read "CAN 通道"() -> (w585:u32)
        n483 = local read "设备类型"() -> (w583:u32)
        n484 = local read "索引"() -> (w584:u32)
        n485 = dll-call lib="PTH1?abs E源码LV源码CAN\nCAN_ZLG3.7CANControlCAN.dll" fn="VCI_StartCAN"("DeviceType"=w583, "DeviceInd"=w584, "CANInd"=w585) -> ("返回类型"=w586:u32)  [unwired: 6 in, 2 out]
        n486 = Equal?(x=w586, y=u32 1) -> (x = y?=w588:bool)
        n487 = case shown="真" w588 {
          selector: w588 -> [_ w590]
          frame False {
          }
          frame True {
            w589 = 2
            n488 = property on="索引" class="Ring (严格)"("DisabledEnum"=w589) -> ()  [unwired: 2 in, 2 out]
            n489 = property on="CAN 通道" class="Ring (严格)"("DisabledEnum"=w589) -> ()  [unwired: 2 in, 2 out]
            "CANStartup" <- w590
          }
        }
      }
      event "ResetCAN": Value Change {
        n490 = event-data() -> ()  [unwired: 1 in, 6 out]
        n491 = local read "CAN 通道"() -> (w593:u32)
        n492 = local read "设备类型"() -> (w591:u32)
        n493 = local read "索引"() -> (w592:u32)
        n494 = dll-call lib="PTH1?abs E源码LV源码CAN\nCAN_ZLG3.7CANControlCAN.dll" fn="VCI_ResetCAN"("DeviceType"=w591, "DeviceInd"=w592, "CANInd"=w593) -> (w594:u32)  [unwired: 6 in, 2 out]
        n495 = Equal?(x=w594, y=u32 1) -> (x = y?=w597:bool)
        n496 = case shown="真" w597 {
          frame False {
          }
          frame True {
            w598 = T39."Enabled" ("禁用")
            n497 = property on="索引" class="Ring (严格)"("DisabledEnum"=w598) -> ()  [unwired: 2 in, 2 out]
            n498 = property on="CAN 通道" class="Ring (严格)"("DisabledEnum"=w598) -> ()  [unwired: 2 in, 2 out]
          }
        }
        n499 = local write "CANStartup"(FALSE) -> ()
      }
      event "HVAC请求信号开关": Value Change {
        n500 = event-data() -> ("NewVal"=w602:bool)  [unwired: 1 in]
        n501 = Unbundle By Name(w601) -> ("空调开启状态"=w600:refnum<vi>)
        n502 = property class="Bool (严格)"(reference=w600, "Value"=w602) -> ()  [unwired: 1 in, 2 out]
      }
      event "空调开启状态": Value Change {
        n503 = event-data() -> ("NewVal"=w605:bool)  [unwired: 1 in]
        n504 = Unbundle By Name(w604) -> ("HVAC请求信号开关"=w603:refnum<vi>)
        n505 = property class="Bool (严格)"(reference=w603, "Value"=w605) -> ()  [unwired: 1 in, 2 out]
      }
      event Panel Close? {
        n506 = event-data() -> ()  [unwired: 1 in, 4 out]
        n507 = Two Button Dialog(message="程序正在运行确定退出？" ("消息")) -> (T button?=w607:bool)  [unwired: 2 in]
        n508 = case shown="真" w607 {
          tunnel: [_ w610] -> w606
          frame False {
          }
          frame True {
            n509 = stacked-sequence {
              tunnel: [_ _ w615] -> w610
              frame #0 {
                n510 = local read "设备类型"() -> (w611:u32)
                n511 = dll-call lib="PTH1?abs E源码LV源码CAN\nCAN_ZLG3.7CANControlCAN.dll" fn="VCI_CloseDevice"("DeviceType"=w611, "DeviceInd"=0) -> ()  [unwired: 5 in, 3 out]
              }
              frame #1 {
                # "这个延时必须要"
                n512 = property on="设备类型" class="Ring (严格)"("DisabledEnum"=T39."Enabled" ("禁用")) -> ()  [unwired: 2 in, 2 out]
                n513 = Wait (ms)(milliseconds to wait=u32 500 ("等待时间（毫秒）")) -> ()  [unwired: 1 out]
              }
              frame #2 {
                w615 = TRUE
                n514 = global write "GlobalVariable.vi" "Exit"(w615) -> ()
              }
            }
            n515 = local write "CANStartup"(FALSE) -> ()
          }
        }
        n516 = event-data("Discard?"=w607) -> ()  [unwired: 1 in, 1 out]
      }
      event Timeout {
        w638 = u32 0
        w625 = u32 0
        n517 = event-data() -> ()  [unwired: 1 in, 3 out]
        n518 = call "CurrentTime.vi"("Input1"=w616) -> ()  [unwired: 10 in, 1 out]
        n519 = for {
          N: 8 -> [_]
          tunnel: "数据输入" -> [w662]
          tunnel: [w665] -> w622 mode=indexing
          tunnel: [w650] -> w629
          i -> [w655]
          n520 = Multiply(x=3, y=w655) -> (x*y=w668:i32)
          n521 = String Length(string=w662) -> (length=w661:i32)
          n522 = String Subset(string=w662, offset (0)=w668, length (rest)=2 ("length (rest)")) -> (substring=w659:string)
          n523 = Quotient & Remainder(x=w661, y=3) -> (x-y*floor(x/y)=w657:i32, floor(x/y)=w653:i32)
          n524 = Equal To 0?(x=w657) -> (x = 0?=w656:bool)
          n525 = Increment(x=w653) -> (x+1=w654:i32)
          n526 = Hex Digit?(1:w659) -> (0:w663:bool)
          n527 = Select(t=w653, s=w656, f=w654) -> (s? t:f=w652:i32)
          n528 = Select(t=w659, s=w663, f="00" ("t")) -> (s? t:f=w664:string)
          n529 = Quotient & Remainder(x=w652, y=9) -> (x-y*floor(x/y)=w650:i32)  [unwired: 1 out]
          n530 = Scan From String(format string="%2x ", input string=w664) -> (output 1=w665:u32)  [unwired: 2 in, 4 out]
        }
        n531 = Bundle("验收码"="验收码", "屏蔽码"="屏蔽码", 0, "滤波方式"="滤波方式", "BTR0"="BTR0", "BTR1"="BTR1", "模式"="模式") -> (→"VCI_INIT_CONFIG":T40)  [unwired: 1 in]
        n532 = Array To Cluster(array=w622) -> (cluster=w623:T41)
        n533 = local read "CAN 通道"() -> (w619:u32)
        n534 = Unbundle(w623) -> ("[0]"=w630:u32, "[1]"=w631:u32, "[2]"=w632:u32, "[3]"=w633:u32, "[4]"=w634:u32, "[5]"=w635:u32, "[6]"=w636:u32, "[7]"=w637:u32)  [unwired: 1 out]
        n535 = local read "设备类型"() -> (w640:u32)
        n536 = local read "索引"() -> (w641:u32)
        n537 = To Unsigned Byte Integer(number=w625) -> (unsigned 8bit integer=w624:u8)
        n538 = dll-call lib="PTH1?abs E源码LV源码CAN\nCAN_ZLG3.7CANControlCAN.dll" fn="VCI_GetReceiveNum"("DeviceType"=w640, "DeviceInd"=w641, "CANInd"=w619) -> ("返回类型"=→"接收缓冲区":u32)  [unwired: 6 in, 2 out]
        n539 = Bundle("发送 ID"="发送 ID", w625, w624, "发送类型"="发送类型", "帧格式"="帧格式", "帧类型"="帧类型", w629, "[0]"=w630, "[1]"=w631, "[2]"=w632, "[3]"=w633, "[4]"=w634, "[5]"=w635, "[6]"=w636, "[7]"=w637, w638, w638, w638) -> (→"VCI_CAN_OBJ_T":T42)  [unwired: 1 in]
      }
    }
  }
  n540 = while {
    tunnel: w7 -> [w686]
    tunnel: w8 -> [w683]
    tunnel: w3 -> [w682]
    shift-right: [w681] -> w14
    shift-left: T23 {"TCU档位模式"=0, "仪表显示档位状态"=0} ("TCU") -> [w680]
    shift-right: [w677] -> _
    shift-left: T22 {"ESC信号提示ESP失败"=FALSE, "ABS_ESC信号提示车速有效性"=FALSE, "ABS_ESC信号提示车速"=0.0, "AVH提示状态"=0, "EPB系统错误指示"=FALSE, "提示HHC功能是否失效"=FALSE} ("ESC状态") -> [w679]
    tunnel: w5 -> [w678]
    tunnel: w6 -> [w676]
    i -> [w673]
    stop <- w685 stop-if-true
    # "周期20ms主动发送类ID"
    n541 = local read "CANStartup"() -> (w684:bool)
    n542 = case shown="无错误" w686 {
      selector: w686 -> [w687 w806]
      tunnel: w684 -> [w701 _]
      tunnel: w683 -> [w700 _]
      tunnel: w682 -> [w699 _]
      tunnel: [w698 w808] -> w681
      tunnel: w680 -> [w697 w808]
      tunnel: w679 -> [w696 w807]
      tunnel: w678 -> [w695 _]
      tunnel: [w694 w807] -> w677
      tunnel: w676 -> [w693 _]
      tunnel: [w688 w806] -> w675
      tunnel: [w692 TRUE ("Exit")] -> w674
      tunnel: w673 -> [w691 _]
      tunnel: "TCU控制:113" -> [w690 _]
      tunnel: "ESC控制:125" -> [w689 _]
      frame No Error {
        n543 = case shown="真" w701 {
          tunnel: w700 -> [_ w729]
          tunnel: w699 -> [_ w728]
          tunnel: [w706 w727] -> w698
          tunnel: w697 -> [w706 _]
          tunnel: w696 -> [w705 w724]
          tunnel: w695 -> [_ w722]
          tunnel: [w705 w718] -> w694
          tunnel: w693 -> [_ w715]
          tunnel: [w704 w712] -> w692
          tunnel: w691 -> [_ w710]
          tunnel: w690 -> [_ w709]
          tunnel: w689 -> [_ w708]
          tunnel: [w702 w707] -> w688
          tunnel: w687 -> [w702 _]
          frame False {
            # "这个延时必须要，不然程序卡在此处"
            n544 = Wait (ms)(milliseconds to wait=u32 2 ("等待时间（毫秒）")) -> ()  [unwired: 1 out]
            n545 = global read "GlobalVariable.vi" "Exit"() -> (w704:bool)
          }
          frame True {
            n546 = flat-sequence {
              tunnel: w729 -> [w763]
              tunnel: w728 -> [w762]
              tunnel: [w759] -> w726
              tunnel: [w749] -> w725
              tunnel: w724 -> [_]
              tunnel: [w748] -> w723
              tunnel: w722 -> [w748]
              tunnel: [w747] -> w721
              tunnel: [w746] -> w720
              tunnel: [w745] -> w719
              tunnel: [w744] -> w717
              tunnel: [w743] -> w716
              tunnel: w715 -> [w743]
              tunnel: [w737] -> w714
              tunnel: [w742] -> w713
              tunnel: [w742] -> w712
              tunnel: [20] -> w711
              tunnel: w710 -> [w739]
              tunnel: w709 -> [w731]
              tunnel: w708 -> [w730]
              tunnel: [w788] -> w727
              tunnel: w726 -> [w788]
              tunnel: w725 -> [w787]
              tunnel: w723 -> [w786]
              tunnel: w721 -> [w785]
              tunnel: w720 -> [w784]
              tunnel: w719 -> [w783]
              tunnel: [w782] -> w718
              tunnel: w717 -> [w782]
              tunnel: w716 -> [w781]
              tunnel: w714 -> [w780]
              tunnel: w713 -> [w778]
              tunnel: w711 -> [w779]
              tunnel: [w777] -> w707
              frame #0 {
                w736 = u32[] [275, 293]
                n547 = call "TCU_113_ctl.vi"("Input2"=w762, "Input1"=w763) -> ("TCU113"=w759:T23, "CmdStr"=w761:string)  [unwired: 7 in, 1 out]
                n548 = call "ESC_125_ctl.vi"("Input2"=w762, "Input1"=w763) -> ("ESC125"=w744:T22, "CmdStr"=w760:string)  [unwired: 7 in, 1 out]
                n549 = local read "发送类型"() -> (w758:u8)
                n550 = Build Array(w761, w760) -> (w757:string[])
                n551 = Build Array(w731, w730) -> (w735:bool[])
                n552 = for {
                  tunnel: w758 -> [w776]
                  tunnel: w757 -> [w775] mode=indexing
                  tunnel: w735 -> [w774] mode=indexing
                  tunnel: w736 -> [w773] mode=indexing
                  tunnel: [w772] -> w756 mode=indexing
                  n553 = call "DataToCANPack.vi"("发送类型"=w776, "数据输入"=w775, "ID"=w773, "启用"=w774) -> ("VCI_CAN_OBJT"=w772:T9)  [unwired: 10 in, 1 out]
                }
                n554 = call "ArrayConstant.vi"() -> ("VCI_CAN_OBJ_RN"=w755:T7)
                n555 = To Unsigned Byte Integer(number=w739) -> (unsigned 8bit integer=w738:u8)
                n556 = call "StrMissingCount.vi"("BoolCtl"=w735, "IDStrIn"=w736) -> ("StrOut"=w734:string)  [unwired: 8 in, 1 out]
                n557 = for {
                  tunnel: w735 -> [w767] mode=indexing
                  tunnel: w756 -> [w765] mode=indexing
                  shift-right: [w764] -> w746
                  shift-left: w755 -> [w766]
                  n558 = case shown="真" w767 {
                    tunnel: w766 -> [w768 w771]
                    tunnel: w765 -> [_ w770]
                    tunnel: [w768 w769] -> w764
                    frame False {
                    }
                    frame True {
                      n559 = Insert Into Array(array=w771, new element=w770) -> (w769:T7)  [unwired: 1 in]
                    }
                  }
                }
                n560 = Number To Decimal String(number=w738) -> (decimal integer string=w732:string)  [unwired: 1 in]
                n561 = local read "CAN 通道"() -> (w752:u32)
                n562 = local read "设备类型"() -> (w754:u32)
                n563 = local read "索引"() -> (w753:u32)
                n564 = Array Size(array=w746) -> (size(s)=w751:i32)
                n565 = Concatenate Strings("主动发送ID：", w734, "失败！", w732) -> (w737:string)
                n566 = local read "VCI_CAN_OBJ_T"() -> (w745:T9)
                n567 = To Unsigned Long Integer(number=w751) -> (unsigned 32bit integer=w750:u32)
                n568 = global read "GlobalVariable.vi" "Exit"() -> (w742:bool)
                n569 = dll-call lib="PTH1?abs E源码LV源码CAN\nCAN_ZLG3.7CANControlCAN.dll" fn="VCI_Transmit"("DeviceType"=w754, "DeviceInd"=w753, "CANInd"=w752, "pSend"=w746, "Len"=w751) -> ("return type"=w747:u32)  [unwired: 7 in, 3 out]
                n570 = Greater Or Equal?(x=w747, y=w750) -> (x >= y?=w749:bool)
              }
              frame #1 {
                n571 = case shown="假" w787 {
                  tunnel: w781 -> [_ w803]
                  tunnel: w783 -> [_ w802]
                  tunnel: w785 -> [_ w801]
                  tunnel: w786 -> [w796 _]
                  tunnel: w780 -> [w792 _]
                  tunnel: w784 -> [_ w799]
                  tunnel: w778 -> [_ _]
                  tunnel: [w790 w797] -> w777
                  frame False {
                    n572 = Bundle By Name(cluster=T3 {"Event"="", "Value"=variant} ("Log"), "Event"="Error", "Value"=w792) -> (w794:T3)
                    n573 = Generate User Event(user event=w796, event data cluster=w794) -> (error out=w791:errorcluster)  [unwired: 2 in, 1 out]
                    n574 = call <vilib>:"Clear Errors.vi"("error in (no error)"=w791) -> ("error out"=w790:errorcluster)  [unwired: 6 in]
                  }
                  frame True {
                    n575 = Bundle(TRUE, "VCI_CAN_OBJ_T"=w802, "VCI_CAN_OBJ_RN"=w799, "return type"=w801) -> (w800:T33)  [unwired: 1 in]
                    n576 = Generate User Event(user event=w803, event data cluster=w800) -> (error out=w798:errorcluster)  [unwired: 2 in, 1 out]
                    n577 = call <vilib>:"Clear Errors.vi"("error in (no error)"=w798) -> ("error out"=w797:errorcluster)  [unwired: 6 in]
                  }
                }
                n578 = case shown="假" w778 {
                  tunnel: w779 -> [w789 _]
                  frame False {
                    n579 = Wait (ms)(milliseconds to wait=w789) -> ()  [unwired: 1 out]
                  }
                  frame True {
                  }
                }
              }
            }
          }
        }
      }
      frame Error {
      }
    }
    n580 = global read "GlobalVariable.vi" "Exit"() -> (w672:bool)
    n581 = Compound Arithmetic op=OR(w675, w674, w672) -> (w685:bool)
  }
  n582 = while {
    tunnel: w7 -> [w825]
    tunnel: w8 -> [w823]
    tunnel: w3 -> [w822]
    tunnel: w5 -> [w819]
    tunnel: w6 -> [w818]
    shift-right: [w814] -> w13
    shift-left: T21 {"实际方向盘转向角"=-780.0, "方向盘转角速度"=0, "方向盘转向标定位"=FALSE, "SASFailureStatus"=FALSE, "计数"=0} ("SAS0E0") -> [w815]
    shift-right: [w813] -> _
    shift-left: u16 0 ("Engine_085") -> [w812]
    i -> [w821]
    stop <- w826 stop-if-true
    # "周期10ms主动发送类ID"
    n583 = local read "CANStartup"() -> (w824:bool)
    n584 = To Unsigned Byte Integer(number=w821) -> (unsigned 8bit integer=w820:u8)
    n585 = case shown="无错误" w825 {
      selector: w825 -> [w827 w952]
      tunnel: w824 -> [w842 _]
      tunnel: w823 -> [w841 _]
      tunnel: w822 -> [w840 _]
      tunnel: w820 -> [w839 _]
      tunnel: w819 -> [w838 _]
      tunnel: w818 -> [w837 _]
      tunnel: [w836 TRUE ("Exit")] -> w817
      tunnel: [w828 w952] -> w816
      tunnel: w815 -> [w835 w951]
      tunnel: [w834 w951] -> w814
      tunnel: w812 -> [w833 w950]
      tunnel: [w832 w950] -> w813
      tunnel: w812 -> [w831 _]
      tunnel: "SAS转角状态:0E0" -> [w830 _]
      tunnel: "车机设置:085" -> [w829 _]
      frame No Error {
        n586 = case shown="真" w842 {
          tunnel: w841 -> [_ w872]
          tunnel: w840 -> [_ w871]
          tunnel: w839 -> [_ w870]
          tunnel: w838 -> [_ w868]
          tunnel: w837 -> [_ w862]
          tunnel: [w847 w858] -> w836
          tunnel: w835 -> [w846 w857]
          tunnel: [w846 w856] -> w834
          tunnel: w833 -> [w845 w854]
          tunnel: [w845 w852] -> w832
          tunnel: w831 -> [_ w851]
          tunnel: w830 -> [_ w850]
          tunnel: w829 -> [_ w849]
          tunnel: [w843 w848] -> w828
          tunnel: w827 -> [w843 _]
          frame False {
            # "这个延时必须要，不然程序卡在此处"
            n587 = Wait (ms)(milliseconds to wait=u32 2 ("等待时间（毫秒）")) -> ()  [unwired: 1 out]
            n588 = global read "GlobalVariable.vi" "Exit"() -> (w847:bool)
          }
          frame True {
            n589 = flat-sequence {
              tunnel: w872 -> [w907]
              tunnel: w871 -> [w906]
              tunnel: w870 -> [w905]
              tunnel: [w897] -> w869
              tunnel: w868 -> [w897]
              tunnel: [w894] -> w867
              tunnel: [w893] -> w866
              tunnel: [w892] -> w865
              tunnel: [w891] -> w864
              tunnel: [w890] -> w863
              tunnel: w862 -> [w890]
              tunnel: [w882] -> w861
              tunnel: [w888] -> w860
              tunnel: [10] -> w859
              tunnel: [w888] -> w858
              tunnel: w857 -> [_]
              tunnel: [w887] -> w855
              tunnel: w854 -> [_]
              tunnel: [w886] -> w853
              tunnel: w851 -> [w881]
              tunnel: w850 -> [w874]
              tunnel: w849 -> [w873]
              tunnel: w869 -> [w932]
              tunnel: w867 -> [w931]
              tunnel: w866 -> [w930]
              tunnel: w865 -> [w929]
              tunnel: w864 -> [w928]
              tunnel: w863 -> [w927]
              tunnel: w861 -> [w926]
              tunnel: w860 -> [w922]
              tunnel: w859 -> [w925]
              tunnel: [w924] -> w856
              tunnel: w855 -> [w924]
              tunnel: w853 -> [w923]
              tunnel: [w923] -> w852
              tunnel: [w921] -> w848
              frame #0 {
                w879 = u32[] [224, 133]
                n590 = call "SAS_0E0_ctl.vi"("Input2"=w906, "计数"=w905, "Input1"=w907) -> ("SAS0E0"=w887:T21, "CmdStr"=w904:string)  [unwired: 6 in, 1 out]
                n591 = call "EMS_085_ctl.vi"("Input2"=w906, "Input1"=w907) -> ("Engine_085"=w886:u16, "CmdStr"=w903:string)  [unwired: 7 in, 1 out]
                n592 = local read "发送类型"() -> (w901:u8)
                n593 = Build Array(w904, w903) -> (w902:string[])
                n594 = Build Array(w874, w873) -> (w878:bool[])
                n595 = To Unsigned Byte Integer(number=w881) -> (unsigned 8bit integer=w880:u8)
                n596 = for {
                  tunnel: w901 -> [w920]
                  tunnel: w902 -> [w919] mode=indexing
                  tunnel: w878 -> [w918] mode=indexing
                  tunnel: w879 -> [w917] mode=indexing
                  tunnel: [w916] -> w885 mode=indexing
                  n597 = call "DataToCANPack.vi"("发送类型"=w920, "数据输入"=w919, "ID"=w917, "启用"=w918) -> ("VCI_CAN_OBJT"=w916:T9)  [unwired: 10 in, 1 out]
                }
                n598 = call "ArrayConstant.vi"() -> ("VCI_CAN_OBJ_RN"=w884:T7)
                n599 = call "StrMissingCount.vi"("BoolCtl"=w878, "IDStrIn"=w879) -> ("StrOut"=w877:string)  [unwired: 8 in, 1 out]
                n600 = for {
                  tunnel: w878 -> [w911] mode=indexing
                  tunnel: w885 -> [w909] mode=indexing
                  shift-right: [w908] -> w891
                  shift-left: w884 -> [w910]
                  n601 = case shown="真" w911 {
                    tunnel: w910 -> [w912 w915]
                    tunnel: w909 -> [_ w914]
                    tunnel: [w912 w913] -> w908
                    frame False {
                    }
                    frame True {
                      n602 = Insert Into Array(array=w915, new element=w914) -> (w913:T7)  [unwired: 1 in]
                    }
                  }
                }
                n603 = local read "CAN 通道"() -> (w898:u32)
                n604 = local read "设备类型"() -> (w900:u32)
                n605 = Number To Decimal String(number=w880) -> (decimal integer string=w875:string)  [unwired: 1 in]
                n606 = local read "索引"() -> (w899:u32)
                n607 = Array Size(array=w891) -> (size(s)=w896:i32)
                n608 = Concatenate Strings("主动发送ID：", w877, "失败！", w875) -> (w882:string)
                n609 = local read "VCI_CAN_OBJ_T"() -> (w892:T9)
                n610 = To Unsigned Long Integer(number=w896) -> (unsigned 32bit integer=w895:u32)
                n611 = dll-call lib="PTH1?abs E源码LV源码CAN\nCAN_ZLG3.7CANControlCAN.dll" fn="VCI_Transmit"("DeviceType"=w900, "DeviceInd"=w899, "CANInd"=w898, "pSend"=w891, "Len"=w896) -> ("return type"=w893:u32)  [unwired: 7 in, 3 out]
                n612 = global read "GlobalVariable.vi" "Exit"() -> (w888:bool)
                n613 = Greater Or Equal?(x=w893, y=w895) -> (x >= y?=w894:bool)
              }
              frame #1 {
                n614 = case shown="真" w931 {
                  tunnel: w927 -> [_ w947]
                  tunnel: w929 -> [_ w946]
                  tunnel: w930 -> [_ w945]
                  tunnel: w932 -> [w940 _]
                  tunnel: w926 -> [w936 _]
                  tunnel: w928 -> [_ w943]
                  tunnel: w922 -> [_ _]
                  tunnel: [w934 w941] -> w921
                  frame False {
                    n615 = Bundle By Name(cluster=T3 {"Event"="", "Value"=variant} ("Log"), "Event"="Error", "Value"=w936) -> (w938:T3)
                    n616 = Generate User Event(user event=w940, event data cluster=w938) -> (error out=w935:errorcluster)  [unwired: 2 in, 1 out]
                    n617 = call <vilib>:"Clear Errors.vi"("error in (no error)"=w935) -> ("error out"=w934:errorcluster)  [unwired: 6 in]
                  }
                  frame True {
                    n618 = Bundle(TRUE, "VCI_CAN_OBJ_T"=w946, "VCI_CAN_OBJ_RN"=w943, "return type"=w945) -> (w944:T33)  [unwired: 1 in]
                    n619 = Generate User Event(user event=w947, event data cluster=w944) -> (error out=w942:errorcluster)  [unwired: 2 in, 1 out]
                    n620 = call <vilib>:"Clear Errors.vi"("error in (no error)"=w942) -> ("error out"=w941:errorcluster)  [unwired: 6 in]
                  }
                }
                n621 = case shown="假" w922 {
                  tunnel: w925 -> [w933 _]
                  frame False {
                    n622 = Wait (ms)(milliseconds to wait=w933) -> ()  [unwired: 1 out]
                  }
                  frame True {
                  }
                }
              }
            }
          }
        }
      }
      frame Error {
      }
    }
    n623 = global read "GlobalVariable.vi" "Exit"() -> (w811:bool)
    n624 = Compound Arithmetic op=OR(w816, w817, w811) -> (w826:bool)
  }
  n625 = while {
    tunnel: w5 -> [w964]
    shift-right: [w960] -> w11
    shift-left: T19 {"秒"=0, "分"=0, "时"=0, "时间显示制"=0, "日"=0, "月"=0, "年"=0} ("IPK时间:3F0") -> [w961]
    tunnel: w6 -> [w959]
    tunnel: w7 -> [w957]
    tunnel: w8 -> [w956]
    tunnel: w3 -> [w955]
    i -> [w958]
    stop <- w966 stop-if-true
    # "时间ID：3F0周期发送"
    n626 = local read "CANStartup"() -> (w965:bool)
    n627 = case shown="无错误" w957 {
      selector: w957 -> [w967 w1076]
      tunnel: w965 -> [w978 _]
      tunnel: w964 -> [w977 _]
      tunnel: [w976 TRUE ("Exit")] -> w963
      tunnel: [w968 w1076] -> w962
      tunnel: w961 -> [w975 w1075]
      tunnel: [w974 w1075] -> w960
      tunnel: w959 -> [w973 _]
      tunnel: w958 -> [w972 _]
      tunnel: w956 -> [w971 _]
      tunnel: w955 -> [w970 _]
      tunnel: "IPK时间:3F0" -> [w969 _]
      frame No Error {
        n628 = case shown="真" w978 {
          tunnel: w977 -> [_ w1001]
          tunnel: [w982 w993] -> w976
          tunnel: w975 -> [w981 w992]
          tunnel: [w981 w991] -> w974
          tunnel: w973 -> [_ w989]
          tunnel: w972 -> [_ w988]
          tunnel: w971 -> [_ w987]
          tunnel: w970 -> [_ w986]
          tunnel: w969 -> [_ w984]
          tunnel: [w979 w983] -> w968
          tunnel: w967 -> [w979 _]
          frame False {
            # "这个延时必须要，不然程序卡在此处"
            n629 = Wait (ms)(milliseconds to wait=u32 2 ("等待时间（毫秒）")) -> ()  [unwired: 1 out]
            n630 = global read "GlobalVariable.vi" "Exit"() -> (w982:bool)
          }
          frame True {
            n631 = flat-sequence {
              tunnel: [w1027] -> w1002
              tunnel: w1001 -> [w1027]
              tunnel: [w1024] -> w1000
              tunnel: [w1023] -> w999
              tunnel: [w1022] -> w998
              tunnel: [w1021] -> w997
              tunnel: [w1012] -> w996
              tunnel: [w1019] -> w995
              tunnel: [1000] -> w994
              tunnel: [w1019] -> w993
              tunnel: w992 -> [_]
              tunnel: [w1018] -> w990
              tunnel: w989 -> [w1009]
              tunnel: w988 -> [w1015]
              tunnel: w987 -> [w1011]
              tunnel: w986 -> [w1010]
              tunnel: [w1009] -> w985
              tunnel: w984 -> [w1003]
              tunnel: w1002 -> [w1057]
              tunnel: w1000 -> [w1056]
              tunnel: w999 -> [w1055]
              tunnel: w998 -> [w1054]
              tunnel: w997 -> [w1053]
              tunnel: w996 -> [w1052]
              tunnel: w995 -> [w1049]
              tunnel: w994 -> [w1051]
              tunnel: [w1050] -> w991
              tunnel: w990 -> [w1050]
              tunnel: w985 -> [w1048]
              tunnel: [w1047] -> w983
              frame #0 {
                w1008 = u32[] [1008]
                n632 = call "Time_3F0_ctl.vi"("Input2"=w1010, "Input1"=w1011) -> ("IPK:3F0"=w1018:T19, "CmdStr"=w1033:string)  [unwired: 7 in, 1 out]
                n633 = Build Array(w1003) -> (w1007:bool[])
                n634 = local read "发送类型"() -> (w1031:u8)
                n635 = Build Array(w1033) -> (w1032:string[])
                n636 = for {
                  tunnel: w1031 -> [w1046]
                  tunnel: w1032 -> [w1045] mode=indexing
                  tunnel: w1007 -> [w1042] mode=indexing
                  tunnel: w1008 -> [w1044] mode=indexing
                  tunnel: [w1043] -> w1016 mode=indexing
                  n637 = call "DataToCANPack.vi"("发送类型"=w1046, "数据输入"=w1045, "ID"=w1044, "启用"=w1042) -> ("VCI_CAN_OBJT"=w1043:T9)  [unwired: 10 in, 1 out]
                }
                n638 = call "ArrayConstant.vi"() -> ("VCI_CAN_OBJ_RN"=w1017:T7)
                n639 = To Unsigned Byte Integer(number=w1015) -> (unsigned 8bit integer=w1014:u8)
                n640 = for {
                  tunnel: w1007 -> [w1034] mode=indexing
                  tunnel: w1016 -> [w1036] mode=indexing
                  shift-right: [w1035] -> w1021
                  shift-left: w1017 -> [w1037]
                  n641 = case shown="真" w1034 {
                    tunnel: w1037 -> [w1038 w1041]
                    tunnel: w1036 -> [_ w1040]
                    tunnel: [w1038 w1039] -> w1035
                    frame False {
                    }
                    frame True {
                      n642 = Insert Into Array(array=w1041, new element=w1040) -> (w1039:T7)  [unwired: 1 in]
                    }
                  }
                }
                n643 = call "StrMissingCount.vi"("BoolCtl"=w1007, "IDStrIn"=w1008) -> ("StrOut"=w1006:string)  [unwired: 8 in, 1 out]
                n644 = Number To Decimal String(number=w1014) -> (decimal integer string=w1004:string)  [unwired: 1 in]
                n645 = local read "CAN 通道"() -> (w1028:u32)
                n646 = local read "设备类型"() -> (w1030:u32)
                n647 = local read "索引"() -> (w1029:u32)
                n648 = Array Size(array=w1021) -> (size(s)=w1026:i32)
                n649 = local read "VCI_CAN_OBJ_T"() -> (w1022:T9)
                n650 = To Unsigned Long Integer(number=w1026) -> (unsigned 32bit integer=w1025:u32)
                n651 = dll-call lib="PTH1?abs E源码LV源码CAN\nCAN_ZLG3.7CANControlCAN.dll" fn="VCI_Transmit"("DeviceType"=w1030, "DeviceInd"=w1029, "CANInd"=w1028, "pSend"=w1021, "Len"=w1026) -> ("return type"=w1023:u32)  [unwired: 7 in, 3 out]
                n652 = global read "GlobalVariable.vi" "Exit"() -> (w1019:bool)
                n653 = Concatenate Strings("主动发送ID：", w1006, "失败！", w1004) -> (w1012:string)
                n654 = Greater Or Equal?(x=w1023, y=w1025) -> (x >= y?=w1024:bool)
              }
              frame #1 {
                n655 = case shown="假" w1056 {
                  tunnel: w1054 -> [_ w1072]
                  tunnel: w1055 -> [_ w1071]
                  tunnel: w1057 -> [w1065 _]
                  tunnel: w1052 -> [w1061 _]
                  tunnel: w1053 -> [_ w1069]
                  tunnel: w1049 -> [_ _]
                  tunnel: w1048 -> [_ w1067]
                  tunnel: [w1059 w1066] -> w1047
                  frame False {
                    n656 = Bundle By Name(cluster=T3 {"Event"="", "Value"=variant} ("Log"), "Event"="Error", "Value"=w1061) -> (w1063:T3)
                    n657 = Generate User Event(user event=w1065, event data cluster=w1063) -> (error out=w1060:errorcluster)  [unwired: 2 in, 1 out]
                    n658 = call <vilib>:"Clear Errors.vi"("error in (no error)"=w1060) -> ("error out"=w1059:errorcluster)  [unwired: 6 in]
                  }
                  frame True {
                    n659 = Bundle(TRUE, "VCI_CAN_OBJ_T"=w1072, "VCI_CAN_OBJ_RN"=w1069, "return type"=w1071) -> (w1070:T33)  [unwired: 1 in]
                    n660 = Generate User Event(user event=w1067, event data cluster=w1070) -> (error out=w1068:errorcluster)  [unwired: 2 in, 1 out]
                    n661 = call <vilib>:"Clear Errors.vi"("error in (no error)"=w1068) -> ("error out"=w1066:errorcluster)  [unwired: 6 in]
                  }
                }
                n662 = case shown="假" w1049 {
                  tunnel: w1051 -> [w1058 _]
                  frame False {
                    n663 = Wait (ms)(milliseconds to wait=w1058) -> ()  [unwired: 1 out]
                  }
                  frame True {
                  }
                }
              }
            }
          }
        }
      }
      frame Error {
      }
    }
    n664 = global read "GlobalVariable.vi" "Exit"() -> (w954:bool)
    n665 = Compound Arithmetic op=OR(w962, w963, w954) -> (w966:bool)
  }
  n666 = while {
    tunnel: w6 -> [w1084]
    tunnel: [w1083] -> w31
    tunnel: [w1082] -> w32
    tunnel: w7 -> [w1080]
    stop <- w1081 stop-if-true
    n667 = local read "CANStartup"() -> (w1078:bool)
    n668 = And(x=w1078, y="接收") -> (x .and. y?=w1077:bool)
    n669 = case shown="真" w1077 {
      tunnel: w1084 -> [w1086 w1102]
      tunnel: [w1086 w1101] -> w1083
      tunnel: [w1085 w1100] -> w1082
      tunnel: w1080 -> [w1085 _]
      frame False {
        # "这个延时必须要，不然程序卡在此处"
        n670 = Wait Until Next ms Multiple(millisecond multiple=u32 2 ("毫秒倍数")) -> ()  [unwired: 1 out]
      }
      frame True {
        n671 = local read "设备类型"() -> (w1098:u32)
        n672 = local read "索引"() -> (w1097:u32)
        n673 = local read "CAN 通道"() -> (w1096:u32)
        n674 = local read "VCI_CAN_OBJ_RN"() -> (w1094:T7)
        n675 = dll-call lib="PTH1?abs E源码LV源码CAN\nCAN_ZLG3.7CANControlCAN.dll" fn="VCI_Receive"("DeviceType"=w1098, "DeviceInd"=w1097, "CANInd"=w1096, "pReceive"=w1094, "Len"="arraylen", "WaitTime"=100 ("TimeOut")) -> (error out=w1088:errorcluster, "return type"=w1091:u32, "pReceive"=w1092:T7)  [unwired: 8 in, 1 out]
        n676 = Wait Until Next ms Multiple(millisecond multiple=u32 5 ("毫秒倍数")) -> ()  [unwired: 1 out]
        n677 = local read "VCI_CAN_OBJ_R"() -> (w1103:T9)
        n678 = Greater Or Equal?(x=w1091, y=u32 1) -> (x >= y?=w1089:bool)
        n679 = case shown="真" w1089 {
          tunnel: w1103 -> [_ w1112]
          tunnel: w1102 -> [w1105 w1111]
          tunnel: [w1105 w1110] -> w1101
          tunnel: [w1104 w1109] -> w1100
          tunnel: w1091 -> [_ w1108]
          tunnel: w1092 -> [_ w1107]
          tunnel: w1088 -> [w1104 _]
          frame False {
          }
          frame True {
            n680 = Bundle(FALSE, "VCI_CAN_OBJ_R"=w1112, "pReceive"=w1107, "return type"=w1108) -> (w1106:T43)  [unwired: 1 in]
            n681 = Generate User Event(user event=w1111, event data cluster=w1106) -> (user event out=w1110:refnum<user-event>, error out=w1109:errorcluster)  [unwired: 2 in]
          }
        }
      }
    }
    n682 = global read "GlobalVariable.vi" "Exit"() -> (w1081:bool)
  }
  n683 = while {
    tunnel: w7 -> [w1149]
    shift-right: [w1143] -> w15
    shift-left: T31 {"司机座椅加热状态"=0, "副驾座椅加热状态"=0, "HVSM远程控制模式"=FALSE} ("HVSM") -> [w1144]
    shift-right: [w1139] -> _
    shift-left: T30 {"TCM指示转向灯开关状态"=0, "计数"=0} ("TCM") -> [w1142]
    shift-right: [w1137] -> _
    shift-left: T29 {"HVAC请求信号开关"=FALSE, "AC大气温度传感器合法"=FALSE, "AC大气温度传感器读数"=0.0, "室内空气PM2.5浓度"=0, "室外空气PM2.5浓度"=0, "室内空气质量等级"=0, "PM2.5传感器工作状态"=0, "驻车空调状态"=0, "驻车空调失效状态"=0, "PM2.5是否超标"=FALSE} ("AC命令输入") -> [w1138]
    shift-right: [w1135] -> _
    shift-left: T28 {"自动请求状态"=FALSE, "空调按键引起弹窗显示"=FALSE, "最大制冷请求状态"=FALSE, "除霜请求状态"=FALSE, "内外循环进气"=0, "空气质量传感器请求"=FALSE, "吹风档位"=0, "负离子发生器状态"=0, "吹风模式"=0, "空调开启状态"=FALSE, "左侧设定温度"=18.0, "空调开关按键音"=FALSE, "AC远程控制模式与否"=FALSE, "空调按键触摸状态"=0, "空调按键状态"=0} ("AC命令输入") -> [w1136]
    shift-right: [w1130] -> _
    shift-left: T26 {"驾驶侧车窗有效位"=FALSE, "驾驶侧车窗开度值"=0, "驾驶侧防夹检测"=FALSE, "驾驶侧防夹抑制状态"=FALSE, "驾驶侧车窗运行状态"=0, "驾驶侧车窗位置状态"=0, "驾驶侧车窗故障状态"=FALSE, "左后侧车窗有效位"=FALSE, "左后侧车窗开度值"=0, "左后车窗侧防夹检测"=FALSE, "左后侧车窗防夹抑制状态"=FALSE, "左后侧车窗运行状态"=0, "左后侧车窗位置状态"=0, "左后侧车窗故障状态"=FALSE, "BCM提示左前门状态"=FALSE, "BCM提示左后面状态"=FALSE, "左后门锁状态"=0, "左前门锁状态"=0, "左前门机械钥匙锁止"=FALSE, "后视镜自动折叠应答"=FALSE, "车窗防夹报警应答"=FALSE} ("车身控制命令输入") -> [w1134]
    shift-right: [w1129] -> _
    shift-left: T27 {"后车窗加热器激活"=0, "BCM提示引擎盖开关"=0, "BCM提示后盖箱开关"=FALSE, "后除霜开关"=FALSE, "伴我回家时间选择"=0, "自动开关窗设置"=0, "防盗报警状态"=0, "寻车报警类型设置"=FALSE, "雨刮随速功能"=FALSE, "RLS下雨关窗模式"=0, "智能弯道灯设置"=FALSE, "设防提示类型设置"=0, "日间行车灯设置"=FALSE, "前雨刮激活后雨刮"=FALSE, "手动车是否挂入倒挡"=FALSE, "BCM电源模式"=0, "离合器踏板开关"=FALSE, "车窗透气反馈"=FALSE, "右前盲区可视按键"=FALSE, "天窗/遮阳帘关闭反馈"=FALSE} ("BCM命令输入") -> [w1133]
    shift-right: [w1128] -> _
    shift-left: T25 {"天窗运行状态"=0, "天窗有效位"=FALSE, "天窗水平开度值"=0, "天窗防夹触发"=FALSE, "天窗故障状态"=FALSE, "实际天窗位置"=0} ("BCM命令输入") -> [w1132]
    shift-right: [w1127] -> _
    shift-left: T24 {"PEPS电源模式有效指示"=0, "PEPS电源模式"=0, "PEPS远程在远程模式？"=FALSE, "后备箱不带钥匙解锁配置"=FALSE, "GW信号指示PEPS是否超时1"=FALSE, "GW信号指示PEPS是否超时2"=FALSE, "迎宾灯功能开启关闭响应"=FALSE, "钥匙忘车内锁车报警配置"=FALSE, "电源非OFF锁车报警配置"=FALSE, "任意门开启锁车报警配置"=FALSE} ("GW_PEPS信息") -> [w1131]
    tunnel: w8 -> [w1141]
    tunnel: w3 -> [w1140]
    tunnel: w5 -> [w1126]
    tunnel: w6 -> [w1125]
    i -> [w1124]
    stop <- w1147 stop-if-true
    n684 = local read "CANStartup"() -> (w1148:bool)
    n685 = To Unsigned Byte Integer(number=w1124) -> (unsigned 8bit integer=w1123:u8)
    n686 = case shown="无错误" w1149 {
      selector: w1149 -> [w1159 w1349]
      tunnel: w1148 -> [w1183 _]
      tunnel: [w1150 w1349] -> w1146
      tunnel: [w1182 TRUE] -> w1145
      tunnel: w1144 -> [w1181 w1348]
      tunnel: [w1180 w1348] -> w1143
      tunnel: w1142 -> [w1179 w1347]
      tunnel: w1141 -> [w1178 _]
      tunnel: w1140 -> [w1177 _]
      tunnel: [w1176 w1347] -> w1139
      tunnel: w1138 -> [w1175 w1346]
      tunnel: [w1174 w1346] -> w1137
      tunnel: w1136 -> [w1173 w1345]
      tunnel: [w1172 w1345] -> w1135
      tunnel: w1134 -> [w1171 w1344]
      tunnel: w1133 -> [w1170 w1343]
      tunnel: w1132 -> [w1169 w1342]
      tunnel: w1131 -> [w1168 w1341]
      tunnel: [w1167 w1344] -> w1130
      tunnel: [w1166 w1343] -> w1129
      tunnel: [w1165 w1342] -> w1128
      tunnel: [w1164 w1341] -> w1127
      tunnel: w1126 -> [w1163 _]
      tunnel: w1125 -> [w1162 _]
      tunnel: w1123 -> [w1161 _]
      tunnel: w1123 -> [w1160 _]
      tunnel: "HVSM控制:2C1" -> [w1158 _]
      tunnel: "TCM开关:281" -> [w1157 _]
      tunnel: "AC控制:2F1" -> [w1156 _]
      tunnel: "AC控制:2F2" -> [w1155 _]
      tunnel: "车身控制车窗:285" -> [w1154 _]
      tunnel: "BCM控制:284" -> [w1153 _]
      tunnel: "BCM控制:287" -> [w1152 _]
      tunnel: "车机设置:2FC" -> [w1151 _]
      frame No Error {
        n687 = case shown="真" w1183 {
          tunnel: [w1186 w1218] -> w1182
          tunnel: w1181 -> [w1194 _]
          tunnel: [w1194 w1234] -> w1180
          tunnel: w1179 -> [w1193 _]
          tunnel: w1178 -> [_ w1236]
          tunnel: w1177 -> [_ w1235]
          tunnel: [w1193 w1233] -> w1176
          tunnel: w1175 -> [w1192 _]
          tunnel: [w1192 w1232] -> w1174
          tunnel: w1173 -> [w1191 _]
          tunnel: [w1191 w1231] -> w1172
          tunnel: w1171 -> [w1190 _]
          tunnel: w1170 -> [w1189 _]
          tunnel: w1169 -> [w1188 _]
          tunnel: w1168 -> [w1187 _]
          tunnel: [w1190 w1230] -> w1167
          tunnel: [w1189 w1229] -> w1166
          tunnel: [w1188 w1228] -> w1165
          tunnel: [w1187 w1227] -> w1164
          tunnel: w1163 -> [_ w1216]
          tunnel: w1162 -> [_ w1212]
          tunnel: w1161 -> [_ w1207]
          tunnel: w1160 -> [_ w1206]
          tunnel: w1159 -> [w1184 w1205]
          tunnel: w1158 -> [_ w1204]
          tunnel: w1157 -> [_ w1203]
          tunnel: w1156 -> [_ w1202]
          tunnel: w1155 -> [_ w1201]
          tunnel: w1154 -> [_ w1200]
          tunnel: w1153 -> [_ w1199]
          tunnel: w1152 -> [_ w1198]
          tunnel: w1151 -> [_ w1197]
          tunnel: [w1184 w1196] -> w1150
          frame False {
            # "这个延时必须要，不然程序卡在此处"
            n688 = Wait (ms)(milliseconds to wait=u32 2 ("等待时间（毫秒）")) -> ()  [unwired: 1 out]
            n689 = global read "GlobalVariable.vi" "Exit"() -> (w1186:bool)
          }
          frame True {
            n690 = flat-sequence {
              tunnel: w1236 -> [w1289]
              tunnel: w1235 -> [w1288]
              tunnel: [w1287] -> w1226
              tunnel: [w1286] -> w1225
              tunnel: [w1277] -> w1224
              tunnel: [w1274] -> w1223
              tunnel: [w1273] -> w1222
              tunnel: [w1272] -> w1221
              tunnel: [w1271] -> w1220
              tunnel: [w1270] -> w1219
              tunnel: [w1257] -> w1218
              tunnel: [w1262] -> w1217
              tunnel: [w1261] -> w1215
              tunnel: [w1260] -> w1214
              tunnel: [w1259] -> w1213
              tunnel: w1212 -> [w1258]
              tunnel: [w1258] -> w1211
              tunnel: [w1253] -> w1210
              tunnel: [w1257] -> w1209
              tunnel: [100] -> w1208
              tunnel: w1207 -> [w1255]
              tunnel: w1206 -> [w1252]
              tunnel: w1205 -> [w1238]
              tunnel: w1204 -> [w1246]
              tunnel: w1203 -> [w1245]
              tunnel: w1202 -> [w1244]
              tunnel: w1201 -> [w1243]
              tunnel: w1200 -> [w1242]
              tunnel: w1199 -> [w1241]
              tunnel: w1198 -> [w1240]
              tunnel: w1197 -> [w1239]
              tunnel: [w1237] -> w1195
              tunnel: [w1315] -> w1227
              tunnel: [w1316] -> w1228
              tunnel: [w1317] -> w1229
              tunnel: [w1314] -> w1230
              tunnel: [w1318] -> w1231
              tunnel: [w1319] -> w1232
              tunnel: [w1320] -> w1233
              tunnel: [w1321] -> w1234
              tunnel: w1226 -> [w1321]
              tunnel: w1225 -> [w1320]
              tunnel: w1224 -> [w1319]
              tunnel: w1223 -> [w1318]
              tunnel: w1222 -> [w1314]
              tunnel: w1221 -> [w1317]
              tunnel: w1220 -> [w1316]
              tunnel: w1219 -> [w1315]
              tunnel: w1217 -> [w1313]
              tunnel: w1216 -> [w1312]
              tunnel: w1215 -> [w1311]
              tunnel: w1214 -> [w1310]
              tunnel: w1213 -> [w1309]
              tunnel: w1211 -> [w1308]
              tunnel: w1210 -> [w1307]
              tunnel: w1209 -> [w1305]
              tunnel: w1208 -> [w1306]
              tunnel: [w1304] -> w1196
              tunnel: w1195 -> [w1303]
              frame #0 {
                w1251 = u32[] [705, 641, 753, 754, 645, 644, 647, 764]
                n691 = call "HVSM_ctl.vi"("Input2"=w1288, "Input1"=w1289) -> ("HVSM"=w1287:T31, "CmdStr"=w1285:string)  [unwired: 7 in, 1 out]
                n692 = call "TCM_ctl.vi"("Input2"=w1288, "计数"=w1255, "Input1"=w1289) -> ("TCM"=w1286:T30, "CmdStr"=w1284:string)  [unwired: 6 in, 1 out]
                n693 = call "AC_2F1_ctl.vi"("Input2"=w1288, "Input1"=w1289) -> ("AC2F1"=w1277:T29, "CmdStr"=w1283:string)  [unwired: 7 in, 1 out]
                n694 = call "AC_2F2_ctl.vi"("Input2"=w1288, "Input1"=w1289) -> ("AC2F2"=w1274:T28, "CmdStr"=w1282:string)  [unwired: 7 in, 1 out]
                n695 = call "BCM_285_ctl.vi"("Input2"=w1288, "Input1"=w1289) -> ("BCM285"=w1273:T26, "CmdStr"=w1281:string)  [unwired: 7 in, 1 out]
                n696 = call "BCM_284_ctl.vi"("Input2"=w1288, "Input1"=w1289) -> ("BCM284"=w1272:T27, "CmdStr"=w1280:string)  [unwired: 7 in, 1 out]
                n697 = call "BCM_287_ctl.vi"("Input2"=w1288, "Input1"=w1289) -> ("BCM287"=w1271:T25, "CmdStr"=w1279:string)  [unwired: 7 in, 1 out]
                n698 = call "GW_2FC_ctl.vi"("Input2"=w1288, "Input1"=w1289) -> ("GW2FC"=w1270:T24, "CmdStr"=w1278:string)  [unwired: 7 in, 1 out]
                n699 = Build Array(w1285, w1284, w1283, w1282, w1281, w1280, w1279, w1278) -> (w1275:string[])
                n700 = Build Array(w1246, w1245, w1244, w1243, w1242, w1241, w1240, w1239) -> (w1250:bool[])
                n701 = local read "发送类型"() -> (w1276:u8)
                n702 = for {
                  tunnel: w1276 -> [w1302]
                  tunnel: w1275 -> [w1301] mode=indexing
                  tunnel: w1250 -> [w1300] mode=indexing
                  tunnel: w1251 -> [w1299] mode=indexing
                  tunnel: [w1298] -> w1269 mode=indexing
                  n703 = call "DataToCANPack.vi"("发送类型"=w1302, "数据输入"=w1301, "ID"=w1299, "启用"=w1300) -> ("VCI_CAN_OBJT"=w1298:T9)  [unwired: 10 in, 1 out]
                }
                n704 = call "ArrayConstant.vi"() -> ("VCI_CAN_OBJ_RN"=w1268:T7)
                n705 = call "StrMissingCount.vi"("BoolCtl"=w1250, "IDStrIn"=w1251) -> ("StrOut"=w1249:string)  [unwired: 8 in, 1 out]
                n706 = for {
                  tunnel: w1250 -> [w1293] mode=indexing
                  tunnel: w1269 -> [w1291] mode=indexing
                  shift-right: [w1290] -> w1259
                  shift-left: w1268 -> [w1292]
                  n707 = case shown="真" w1293 {
                    tunnel: w1292 -> [w1294 w1297]
                    tunnel: w1291 -> [_ w1296]
                    tunnel: [w1294 w1295] -> w1290
                    frame False {
                    }
                    frame True {
                      n708 = Insert Into Array(array=w1297, new element=w1296) -> (w1295:T7)  [unwired: 1 in]
                    }
                  }
                }
                n709 = local read "CAN 通道"() -> (w1263:u32)
                n710 = local read "设备类型"() -> (w1265:u32)
                n711 = local read "索引"() -> (w1264:u32)
                n712 = Array Size(array=w1259) -> (size(s)=w1267:i32)
                n713 = local read "VCI_CAN_OBJ_T"() -> (w1260:T9)
                n714 = global read "GlobalVariable.vi" "Exit"() -> (w1257:bool)
                n715 = Number To Decimal String(number=w1252) -> (decimal integer string=w1247:string)  [unwired: 1 in]
                n716 = To Unsigned Long Integer(number=w1267) -> (unsigned 32bit integer=w1266:u32)
                n717 = dll-call lib="PTH1?abs E源码LV源码CAN\nCAN_ZLG3.7CANControlCAN.dll" fn="VCI_Transmit"(error in=w1238, "DeviceType"=w1265, "DeviceInd"=w1264, "CANInd"=w1263, "pSend"=w1259, "Len"=w1267) -> (error out=w1237:errorcluster, "return type"=w1261:u32)  [unwired: 6 in, 2 out]
                n718 = Concatenate Strings("主动发送ID：", w1249, "失败！", w1247) -> (w1253:string)
                n719 = Greater Or Equal?(x=w1261, y=w1266) -> (x >= y?=w1262:bool)
              }
              frame #1 {
                n720 = case shown="真" w1313 {
                  tunnel: w1308 -> [_ w1338]
                  tunnel: w1310 -> [_ w1337]
                  tunnel: w1311 -> [_ w1336]
                  tunnel: w1312 -> [w1330 _]
                  tunnel: w1307 -> [w1326 _]
                  tunnel: w1309 -> [_ w1334]
                  tunnel: w1305 -> [_ _]
                  tunnel: [w1323 w1331] -> w1304
                  tunnel: w1303 -> [w1324 w1332]
                  frame False {
                    n721 = Bundle By Name(cluster=T3 {"Event"="", "Value"=variant} ("Log"), "Event"="Error", "Value"=w1326) -> (w1328:T3)
                    n722 = Generate User Event(user event=w1330, event data cluster=w1328, error in=w1324) -> (error out=w1325:errorcluster)  [unwired: 1 in, 1 out]
                    n723 = call <vilib>:"Clear Errors.vi"("error in (no error)"=w1325) -> ("error out"=w1323:errorcluster)  [unwired: 6 in]
                  }
                  frame True {
                    n724 = Bundle(TRUE, "VCI_CAN_OBJ_T"=w1337, "VCI_CAN_OBJ_RN"=w1334, "return type"=w1336) -> (w1335:T33)  [unwired: 1 in]
                    n725 = Generate User Event(user event=w1338, event data cluster=w1335, error in=w1332) -> (error out=w1333:errorcluster)  [unwired: 1 in, 1 out]
                    n726 = call <vilib>:"Clear Errors.vi"("error in (no error)"=w1333) -> ("error out"=w1331:errorcluster)  [unwired: 6 in]
                  }
                }
                n727 = case shown="假" w1305 {
                  tunnel: w1306 -> [w1322 _]
                  frame False {
                    n728 = Wait (ms)(milliseconds to wait=w1322) -> ()  [unwired: 1 out]
                  }
                  frame True {
                  }
                }
              }
            }
          }
        }
      }
      frame Error {
      }
    }
    n729 = global read "GlobalVariable.vi" "Exit"() -> (w1122:bool)
    n730 = Compound Arithmetic op=OR(w1146, w1145, w1122) -> (w1147:bool)
  }
  n731 = while {
    tunnel: w5 -> [w1361]
    tunnel: w6 -> [w1360]
    shift-right: [w1356] -> w12
    shift-left: T20 {"车窗防夹报警设置应答"=FALSE, "BCM指示转向拔杆状态"=0, "BCM提醒用户位置灯状态"=FALSE} ("BCM_Light") -> [w1357]
    tunnel: w8 -> [w1355]
    tunnel: w3 -> [w1354]
    tunnel: w7 -> [w1353]
    i -> [w1352]
    stop <- w1363 stop-if-true
    # "周期50ms主动发送类ID"
    n732 = local read "CANStartup"() -> (w1362:bool)
    n733 = case shown="无错误" w1353 {
      selector: w1353 -> [w1364 w1473]
      tunnel: w1362 -> [w1375 _]
      tunnel: w1361 -> [w1374 _]
      tunnel: w1360 -> [w1373 _]
      tunnel: [w1372 TRUE ("Exit")] -> w1359
      tunnel: [w1365 w1473] -> w1358
      tunnel: w1357 -> [w1371 w1472]
      tunnel: [w1370 w1472] -> w1356
      tunnel: w1355 -> [w1369 _]
      tunnel: w1354 -> [w1368 _]
      tunnel: w1352 -> [w1367 _]
      tunnel: "车机设置:1F0" -> [w1366 _]
      frame No Error {
        n734 = case shown="真" w1375 {
          tunnel: w1374 -> [_ w1398]
          tunnel: w1373 -> [_ w1392]
          tunnel: [w1379 w1388] -> w1372
          tunnel: w1371 -> [w1378 w1387]
          tunnel: [w1378 w1386] -> w1370
          tunnel: w1369 -> [_ w1384]
          tunnel: w1368 -> [_ w1383]
          tunnel: w1367 -> [_ w1382]
          tunnel: w1366 -> [_ w1381]
          tunnel: [w1376 w1380] -> w1365
          tunnel: w1364 -> [w1376 _]
          frame False {
            # "这个延时必须要，不然程序卡在此处"
            n735 = Wait (ms)(milliseconds to wait=u32 2 ("等待时间（毫秒）")) -> ()  [unwired: 1 out]
            n736 = global read "GlobalVariable.vi" "Exit"() -> (w1379:bool)
          }
          frame True {
            n737 = flat-sequence {
              tunnel: [w1424] -> w1399
              tunnel: w1398 -> [w1424]
              tunnel: [w1421] -> w1397
              tunnel: [w1420] -> w1396
              tunnel: [w1419] -> w1395
              tunnel: [w1418] -> w1394
              tunnel: [w1417] -> w1393
              tunnel: w1392 -> [w1417]
              tunnel: [w1406] -> w1391
              tunnel: [w1415] -> w1390
              tunnel: [50] -> w1389
              tunnel: [w1415] -> w1388
              tunnel: w1387 -> [_]
              tunnel: [w1414] -> w1385
              tunnel: w1384 -> [w1413]
              tunnel: w1383 -> [w1412]
              tunnel: w1382 -> [w1409]
              tunnel: w1381 -> [w1400]
              tunnel: w1399 -> [w1454]
              tunnel: w1397 -> [w1453]
              tunnel: w1396 -> [w1452]
              tunnel: w1395 -> [w1451]
              tunnel: w1394 -> [w1450]
              tunnel: w1393 -> [w1449]
              tunnel: w1391 -> [w1448]
              tunnel: w1390 -> [w1445]
              tunnel: w1389 -> [w1447]
              tunnel: [w1446] -> w1386
              tunnel: w1385 -> [w1446]
              tunnel: [w1444] -> w1380
              frame #0 {
                w1405 = u32[] [496]
                n738 = call "BCM_1F0_ctl.vi"("Input2"=w1412, "Input1"=w1413) -> ("BCM1F0"=w1414:T20, "CmdStr"=w1430:string)  [unwired: 7 in, 1 out]
                n739 = Build Array(w1400) -> (w1404:bool[])
                n740 = local read "发送类型"() -> (w1428:u8)
                n741 = Build Array(w1430) -> (w1429:string[])
                n742 = for {
                  tunnel: w1428 -> [w1443]
                  tunnel: w1429 -> [w1442] mode=indexing
                  tunnel: w1404 -> [w1439] mode=indexing
                  tunnel: w1405 -> [w1441] mode=indexing
                  tunnel: [w1440] -> w1410 mode=indexing
                  n743 = call "DataToCANPack.vi"("发送类型"=w1443, "数据输入"=w1442, "ID"=w1441, "启用"=w1439) -> ("VCI_CAN_OBJT"=w1440:T9)  [unwired: 10 in, 1 out]
                }
                n744 = call "ArrayConstant.vi"() -> ("VCI_CAN_OBJ_RN"=w1411:T7)
                n745 = To Unsigned Byte Integer(number=w1409) -> (unsigned 8bit integer=w1408:u8)
                n746 = for {
                  tunnel: w1404 -> [w1431] mode=indexing
                  tunnel: w1410 -> [w1433] mode=indexing
                  shift-right: [w1432] -> w1418
                  shift-left: w1411 -> [w1434]
                  n747 = case shown="假" w1431 {
                    tunnel: w1434 -> [w1435 w1438]
                    tunnel: w1433 -> [_ w1437]
                    tunnel: [w1435 w1436] -> w1432
                    frame False {
                    }
                    frame True {
                      n748 = Insert Into Array(array=w1438, new element=w1437) -> (w1436:T7)  [unwired: 1 in]
                    }
                  }
                }
                n749 = call "StrMissingCount.vi"("BoolCtl"=w1404, "IDStrIn"=w1405) -> ("StrOut"=w1403:string)  [unwired: 8 in, 1 out]
                n750 = Number To Decimal String(number=w1408) -> (decimal integer string=w1401:string)  [unwired: 1 in]
                n751 = local read "CAN 通道"() -> (w1425:u32)
                n752 = local read "设备类型"() -> (w1427:u32)
                n753 = local read "索引"() -> (w1426:u32)
                n754 = Array Size(array=w1418) -> (size(s)=w1423:i32)
                n755 = local read "VCI_CAN_OBJ_T"() -> (w1419:T9)
                n756 = To Unsigned Long Integer(number=w1423) -> (unsigned 32bit integer=w1422:u32)
                n757 = dll-call lib="PTH1?abs E源码LV源码CAN\nCAN_ZLG3.7CANControlCAN.dll" fn="VCI_Transmit"("DeviceType"=w1427, "DeviceInd"=w1426, "CANInd"=w1425, "pSend"=w1418, "Len"=w1423) -> ("return type"=w1420:u32)  [unwired: 7 in, 3 out]
                n758 = global read "GlobalVariable.vi" "Exit"() -> (w1415:bool)
                n759 = Concatenate Strings("主动发送ID：", w1403, "失败！", w1401) -> (w1406:string)
                n760 = Greater Or Equal?(x=w1420, y=w1422) -> (x >= y?=w1421:bool)
              }
              frame #1 {
                n761 = case shown="假" w1453 {
                  tunnel: w1449 -> [_ w1469]
                  tunnel: w1451 -> [_ w1468]
                  tunnel: w1452 -> [_ w1467]
                  tunnel: w1454 -> [w1462 _]
                  tunnel: w1448 -> [w1458 _]
                  tunnel: w1450 -> [_ w1465]
                  tunnel: w1445 -> [_ _]
                  tunnel: [w1456 w1463] -> w1444
                  frame False {
                    n762 = Bundle By Name(cluster=T3 {"Event"="", "Value"=variant} ("Log"), "Event"="Error", "Value"=w1458) -> (w1460:T3)
                    n763 = Generate User Event(user event=w1462, event data cluster=w1460) -> (error out=w1457:errorcluster)  [unwired: 2 in, 1 out]
                    n764 = call <vilib>:"Clear Errors.vi"("error in (no error)"=w1457) -> ("error out"=w1456:errorcluster)  [unwired: 6 in]
                  }
                  frame True {
                    n765 = Bundle(TRUE, "VCI_CAN_OBJ_T"=w1468, "VCI_CAN_OBJ_RN"=w1465, "return type"=w1467) -> (w1466:T33)  [unwired: 1 in]
                    n766 = Generate User Event(user event=w1469, event data cluster=w1466) -> (error out=w1464:errorcluster)  [unwired: 2 in, 1 out]
                    n767 = call <vilib>:"Clear Errors.vi"("error in (no error)"=w1464) -> ("error out"=w1463:errorcluster)  [unwired: 6 in]
                  }
                }
                n768 = case shown="假" w1445 {
                  tunnel: w1447 -> [w1455 _]
                  frame False {
                    n769 = Wait (ms)(milliseconds to wait=w1455) -> ()  [unwired: 1 out]
                  }
                  frame True {
                  }
                }
              }
            }
          }
        }
      }
      frame Error {
      }
    }
    n770 = global read "GlobalVariable.vi" "Exit"() -> (w1351:bool)
    n771 = Compound Arithmetic op=OR(w1358, w1359, w1351) -> (w1363:bool)
  }
  n772 = while {
    tunnel: w7 -> [w1494]
    tunnel: w6 -> [w1489]
    tunnel: w5 -> [w1488]
    tunnel: [w1474] -> w2
    i -> [w1487]
    stop <- w1491 stop-if-true
    # "丢失类周期发送ID"
    n773 = local read "CANStartup"() -> (w1493:bool)
    n774 = case shown="无错误" w1494 {
      selector: w1494 -> [w1496 w1621]
      tunnel: [w1495 w1621] -> w1492
      tunnel: w1493 -> [w1513 _]
      tunnel: [w1512 TRUE ("Exit")] -> w1490
      tunnel: w1489 -> [w1511 _]
      tunnel: w1488 -> [w1510 w1619]
      tunnel: w1487 -> [w1509 _]
      tunnel: "ICU" -> [w1508 _]
      tunnel: "FCS" -> [w1507 _]
      tunnel: "VCU" -> [w1506 _]
      tunnel: "AVAS" -> [w1505 _]
      tunnel: "TBOX" -> [w1504 _]
      tunnel: "GW" -> [w1503 _]
      tunnel: "PAS" -> [w1502 _]
      tunnel: "DVR" -> [w1501 _]
      tunnel: "SAS" -> [w1500 _]
      tunnel: "OBC" -> [w1499 _]
      tunnel: "BMSH" -> [w1498 _]
      tunnel: [w1497 w1619] -> w1474
      frame No Error {
        n775 = case shown="真" w1513 {
          tunnel: [w1517 w1540] -> w1512
          tunnel: w1511 -> [_ w1538]
          tunnel: w1510 -> [w1515 w1533]
          tunnel: w1509 -> [_ w1531]
          tunnel: w1508 -> [_ w1530]
          tunnel: w1507 -> [_ w1529]
          tunnel: w1506 -> [_ w1528]
          tunnel: w1505 -> [_ w1527]
          tunnel: w1504 -> [_ w1526]
          tunnel: w1503 -> [_ w1525]
          tunnel: w1502 -> [_ w1524]
          tunnel: w1501 -> [_ w1523]
          tunnel: w1500 -> [_ w1522]
          tunnel: w1499 -> [_ w1521]
          tunnel: w1498 -> [_ w1520]
          tunnel: [w1515 w1519] -> w1497
          tunnel: [w1514 w1518] -> w1495
          tunnel: w1496 -> [w1514 _]
          frame False {
            # "这个延时必须要，不然程序卡在此处"
            n776 = Wait (ms)(milliseconds to wait=u32 2 ("等待时间（毫秒）")) -> ()  [unwired: 1 out]
            n777 = global read "GlobalVariable.vi" "Exit"() -> (w1517:bool)
          }
          frame True {
            n778 = flat-sequence {
              tunnel: [100] -> w1542
              tunnel: [w1570] -> w1541
              tunnel: [w1570] -> w1540
              tunnel: [w1567] -> w1539
              tunnel: w1538 -> [w1566]
              tunnel: [w1566] -> w1537
              tunnel: [w1565] -> w1536
              tunnel: [w1564] -> w1535
              tunnel: [w1563] -> w1534
              tunnel: [w1560] -> w1532
              tunnel: w1531 -> [w1561]
              tunnel: w1530 -> [w1553]
              tunnel: w1529 -> [w1552]
              tunnel: w1528 -> [w1551]
              tunnel: w1527 -> [w1549]
              tunnel: w1526 -> [w1548]
              tunnel: w1525 -> [w1547]
              tunnel: w1524 -> [w1546]
              tunnel: w1523 -> [w1545]
              tunnel: w1522 -> [w1544]
              tunnel: w1521 -> [w1550]
              tunnel: w1520 -> [w1543]
              tunnel: w1542 -> [w1600]
              tunnel: w1541 -> [w1591]
              tunnel: w1539 -> [w1599]
              tunnel: w1537 -> [w1598]
              tunnel: w1536 -> [w1597]
              tunnel: w1535 -> [w1596]
              tunnel: w1534 -> [w1595]
              tunnel: w1533 -> [w1594]
              tunnel: w1532 -> [w1593]
              tunnel: [w1592] -> w1519
              tunnel: [w1590] -> w1518
              frame #0 {
                w1558 = u32[] [621, 432, 354, 544, 690, 658, 765, 912, 689, 224, 756]
                n779 = local read "发送类型"() -> (w1577:u8)
                n780 = Build Array(w1553, w1552, w1551, w1550, w1549, w1548, w1547, w1546, w1545, w1544, w1543) -> (w1557:bool[])
                n781 = for {
                  tunnel: [w1589] -> w1576 mode=indexing
                  tunnel: w1577 -> [w1588]
                  tunnel: w1557 -> [w1587] mode=indexing
                  tunnel: w1558 -> [w1586] mode=indexing
                  n782 = call "DataToCANPack.vi"("发送类型"=w1588, "ID"=w1586, "启用"=w1587) -> ("VCI_CAN_OBJT"=w1589:T9)  [unwired: 11 in, 1 out]
                }
                n783 = call "ArrayConstant.vi"() -> ("VCI_CAN_OBJ_RN"=w1575:T7)
                n784 = for {
                  tunnel: w1557 -> [w1581] mode=indexing
                  tunnel: w1576 -> [w1579] mode=indexing
                  shift-right: [w1578] -> w1564
                  shift-left: w1575 -> [w1580]
                  n785 = case shown="真" w1581 {
                    tunnel: w1580 -> [w1582 w1585]
                    tunnel: w1579 -> [_ w1584]
                    tunnel: [w1582 w1583] -> w1578
                    frame False {
                    }
                    frame True {
                      n786 = Insert Into Array(array=w1585, new element=w1584) -> (w1583:T7)  [unwired: 1 in]
                    }
                  }
                }
                n787 = To Unsigned Byte Integer(number=w1561) -> (unsigned 8bit integer=w1559:u8)
                n788 = local read "CAN 通道"() -> (w1572:u32)
                n789 = call "StrMissingCount.vi"("BoolCtl"=w1557, "IDStrIn"=w1558) -> ("StrOut"=w1556:string)  [unwired: 8 in, 1 out]
                n790 = local read "设备类型"() -> (w1574:u32)
                n791 = local read "索引"() -> (w1573:u32)
                n792 = Number To Decimal String(number=w1559) -> (decimal integer string=w1554:string)  [unwired: 1 in]
                n793 = Array Size(array=w1564) -> (size(s)=w1569:i32)
                n794 = local read "VCI_CAN_OBJ_T"() -> (w1565:T9)
                n795 = global read "GlobalVariable.vi" "Exit"() -> (w1570:bool)
                n796 = To Unsigned Long Integer(number=w1569) -> (unsigned 32bit integer=w1568:u32)
                n797 = dll-call lib="PTH1?abs E源码LV源码CAN\nCAN_ZLG3.7CANControlCAN.dll" fn="VCI_Transmit"("DeviceType"=w1574, "DeviceInd"=w1573, "CANInd"=w1572, "pSend"=w1564, "Len"=w1569) -> ("return type"=w1563:u32)  [unwired: 7 in, 3 out]
                n798 = Concatenate Strings("丢失类ID：", w1556, "发送失败！", w1554) -> (w1560:string)
                n799 = Greater Or Equal?(x=w1563, y=w1568) -> (x >= y?=w1567:bool)
              }
              frame #1 {
                n800 = case shown="假" w1599 {
                  tunnel: w1598 -> [_ w1616]
                  tunnel: w1597 -> [_ w1615]
                  tunnel: w1596 -> [_ w1614]
                  tunnel: w1595 -> [_ w1613]
                  tunnel: w1594 -> [w1608 w1610]
                  tunnel: w1593 -> [w1604 _]
                  tunnel: [w1602 w1610] -> w1592
                  tunnel: w1591 -> [_ _]
                  tunnel: [w1601 w1609] -> w1590
                  frame False {
                    n801 = Bundle By Name(cluster=T3 {"Event"="", "Value"=variant} ("Log"), "Event"="Error", "Value"=w1604) -> (w1606:T3)
                    n802 = Generate User Event(user event=w1608, event data cluster=w1606) -> (user event out=w1602:refnum<user-event>, error out=w1603:errorcluster)  [unwired: 2 in]
                    n803 = call <vilib>:"Clear Errors.vi"("error in (no error)"=w1603) -> ("error out"=w1601:errorcluster)  [unwired: 6 in]
                  }
                  frame True {
                    n804 = Bundle(TRUE, "VCI_CAN_OBJ_T"=w1615, "VCI_CAN_OBJ_RN"=w1614, "return type"=w1613) -> (w1612:T33)  [unwired: 1 in]
                    n805 = Generate User Event(user event=w1616, event data cluster=w1612) -> (error out=w1611:errorcluster)  [unwired: 2 in, 1 out]
                    n806 = call <vilib>:"Clear Errors.vi"("error in (no error)"=w1611) -> ("error out"=w1609:errorcluster)  [unwired: 6 in]
                  }
                }
                n807 = case shown="假" w1591 {
                  tunnel: w1600 -> [w1618 _]
                  frame False {
                    n808 = Wait (ms)(milliseconds to wait=w1618) -> ()  [unwired: 1 out]
                  }
                  frame True {
                  }
                }
              }
            }
          }
        }
      }
      frame Error {
      }
    }
    n809 = global read "GlobalVariable.vi" "Exit"() -> (w1486:bool)
    n810 = Compound Arithmetic op=OR(w1492, w1490, w1486) -> (w1491:bool)
  }
  n811 = flat-sequence {
    tunnel: w33 -> [w1635]
    tunnel: w32 -> [w1630]
    tunnel: w31 -> [w1631]
    tunnel: w15 -> [_]
    tunnel: w14 -> [_]
    tunnel: w13 -> [_]
    tunnel: w12 -> [_]
    tunnel: w11 -> [_]
    tunnel: w4 -> [_]
    tunnel: w2 -> [w1626]
    tunnel: w1 -> [_]
    frame #0 {
      n812 = Unregister For Events(event registration refnum=w1635, error in=w1630) -> (error out=w1634:errorcluster)
      n813 = global write "GlobalVariable.vi" "Exit"(FALSE) -> ()
      n814 = global write "GlobalVariable.vi" "Success"(FALSE ("Success")) -> ()
      n815 = Destroy User Event(user event=w1631, error in=w1634) -> (error out=w1629:errorcluster)
      n816 = control-ref of="本VI"() -> (w1625:refnum<vi>)
      n817 = Destroy User Event(user event=w1626, error in=w1629) -> (error out=w1627:errorcluster)
      n818 = global write "GlobalVariable.vi" "列累计"(string[] [] ("列累计")) -> ()
      n819 = invoke class="VI" method="Default Vals.Reinit All"(reference=w1625, error in=w1627) -> (error out=w1624:errorcluster)  [unwired: 1 in, 2 out]
      n820 = property on="OpenDevice" class="Bool (严格)"("BoolText.Text"="打开设备" ("布尔文本.文本")) -> ()  [unwired: 2 in, 2 out]
      n821 = property class="App"(error in=w1624) -> ("App.Kind"=w1632:T44)  [unwired: 1 in, 2 out]
      n822 = case shown="\"Run Time System\"" w1632 {
        frame "invalid app kind", Default {
        }
        frame "Development System" {
        }
        frame "Run Time System" {
          n823 = Quit LabVIEW(quit? (T)=TRUE) -> ()
        }
      }
    }
  }
